vi "运维调试_采配水.vi"() -> ()   [LabVIEW 2016, in "PLC.lvlib"]
uses:
  PLC.lvlib
  <vilib>/Plasmionique/MB Master/MB_Master/MB_Master.lvclass
  <vilib>/Utility/miscctls.llb/LVPointTypeDef.ctl
  <vilib>/Plasmionique/MB Master/MB_Master_Serial/MB_Master_Serial.lvclass
  C:/Program Files (x86)/National Instruments/LabVIEW 2016/vi.lib/Plasmionique/MB Master/MB_Master/MB_Master.lvclass
  <vilib>/Instr/_visa.llb/VISA Configure Serial Port (Instr).vi
  <vilib>/Plasmionique/MB Master/MB Master.lvlib
  <vilib>/ptbypt/NI_PtbyPt.lvlib
panel:
  out "R44":i16
  in  "V14":bool
  in  "看门狗启用":bool
  out "R123":i16 caption="看门狗设置"
  out "R56":i16 caption="看门狗计时器"
  in  "更新程序":bool
  out "R122":i16 caption="二级自来水清洗时间"
  out "R121":i16 caption="一级自来水清洗时间"
  out "R120":i16 caption="过滤自来水清洗时间"
  out "清洗次数":u16
  out "当前启动泵号":u16(ring) items=["1号泵", "2号泵"]
  out "R116":i16 caption="储水时间"
  in  "R113":u16(ring) caption="水箱储水水体" items=["自来水", "水样"]
  out "R112":i16 caption="二级水样池进样超时"
  in  "R111":u16(ring) caption="采配水型号" items=["常规版本", "高配版本"]
  out "数值 19":dbl
  out "数值 18":dbl
  out "数值 17":dbl
  out "数值 16":dbl
  out "数值 15":dbl
  out "数值 14":dbl
  out "数值 13":dbl
  out "数值 12":dbl
  out "数值 11":dbl
  out "数值 10":dbl
  out "数值 9":dbl
  out "数值 8":dbl
  out "数值 7":dbl
  out "数值 6":dbl
  out "数值 5":dbl
  out "数值 4":dbl
  out "数值 3":dbl
  out "数值 2":dbl
  out "数值":dbl
  in  "R118":u16(ring) caption="是否启用质控" items=["不启用质控", "启用质控"]
  out "压力传感器":dbl format="%#.2f"
  out "R110":i16 caption="过滤装置排液时间"
  in  "M4":bool
  in  "M3":bool
  in  "V13":bool
  in  "V12":bool
  in  "V1-R":bool
  in  "V1-G":bool
  in  "V11":bool
  in  "V10":bool
  in  "V9":bool
  in  "V8":bool
  in  "V7-R":bool
  in  "V7-G":bool
  out "X2":bool caption="X1"
  out "采配水版本号":string
  out "R117":i16 caption="清洗频次设定"
  out "通讯故障":bool
  in  "R100":u16(ring) caption="采水泵工作模式" items=["泵1单泵单管路", "泵2单泵单管路", "潜水泵双泵双管路", "自吸泵双泵双管路"]
  out "X11":bool caption="自来水检测_WA"
  out "X10":bool caption="废液报警_WLA"
  out "X9":bool caption="泵2过载报警_KM2"
  out "X8":bool caption="泵1过载报警_KM1"
  out "X7":bool caption="断电检测_DD"
  out "X6":bool caption="门禁开关_MJ"
  out "X5":bool caption="烟雾检测_YW"
  out "X4":bool caption="浸水检测_SJ"
  out "X3":bool caption="水流开关_JY"
  out "X1":bool
  out "X0":bool caption="采样池液位开关_YE1"
  out "R109":i16 caption="外部反冲洗时间"
  out "集成报警信息":string
  out "R108":i16 caption="进样超时时间"
  out "R107":i16 caption="进气时间"
  out "R106":i16 caption="排液时间"
  out "R105":i16 caption="配水时间"
  out "R104":i16 caption="过滤次数"
  out "R103":i16 caption="过滤配水时间"
  out "R102":i16 caption="一级沉淀时间"
  out "R101":i16 caption="管路润洗时间"
  out "R2":i16
  out "R1":i16
  out "多列列表框":i32(listbox)
  in  "V6":bool
  in  "V5":bool
  in  "V4":bool
  in  "V3":bool
  in  "V2":bool
  in  "M2":bool
  in  "M1":bool
  in  "返回":bool
  in  "参数设置":bool
  in  "单步启动":bool
  in  "启动":bool
  in  "停止":bool
  # "流程计时："
  # "s"
  # "压力传感器："
  # "MPa"
  # "二级液位开关低_Y2FD"
  # "二级液位开关高_YF2H"
  # "看门狗设置"
  # "S"
  # "S"
  # "S"
  # "S"
  # "S"
  # "S"
  # "S"
  # "次"
  # "S"
  # "S"
  # "S"
  # "S"
  # "S"
  # "S"
  # "单步计时："
  # "s"
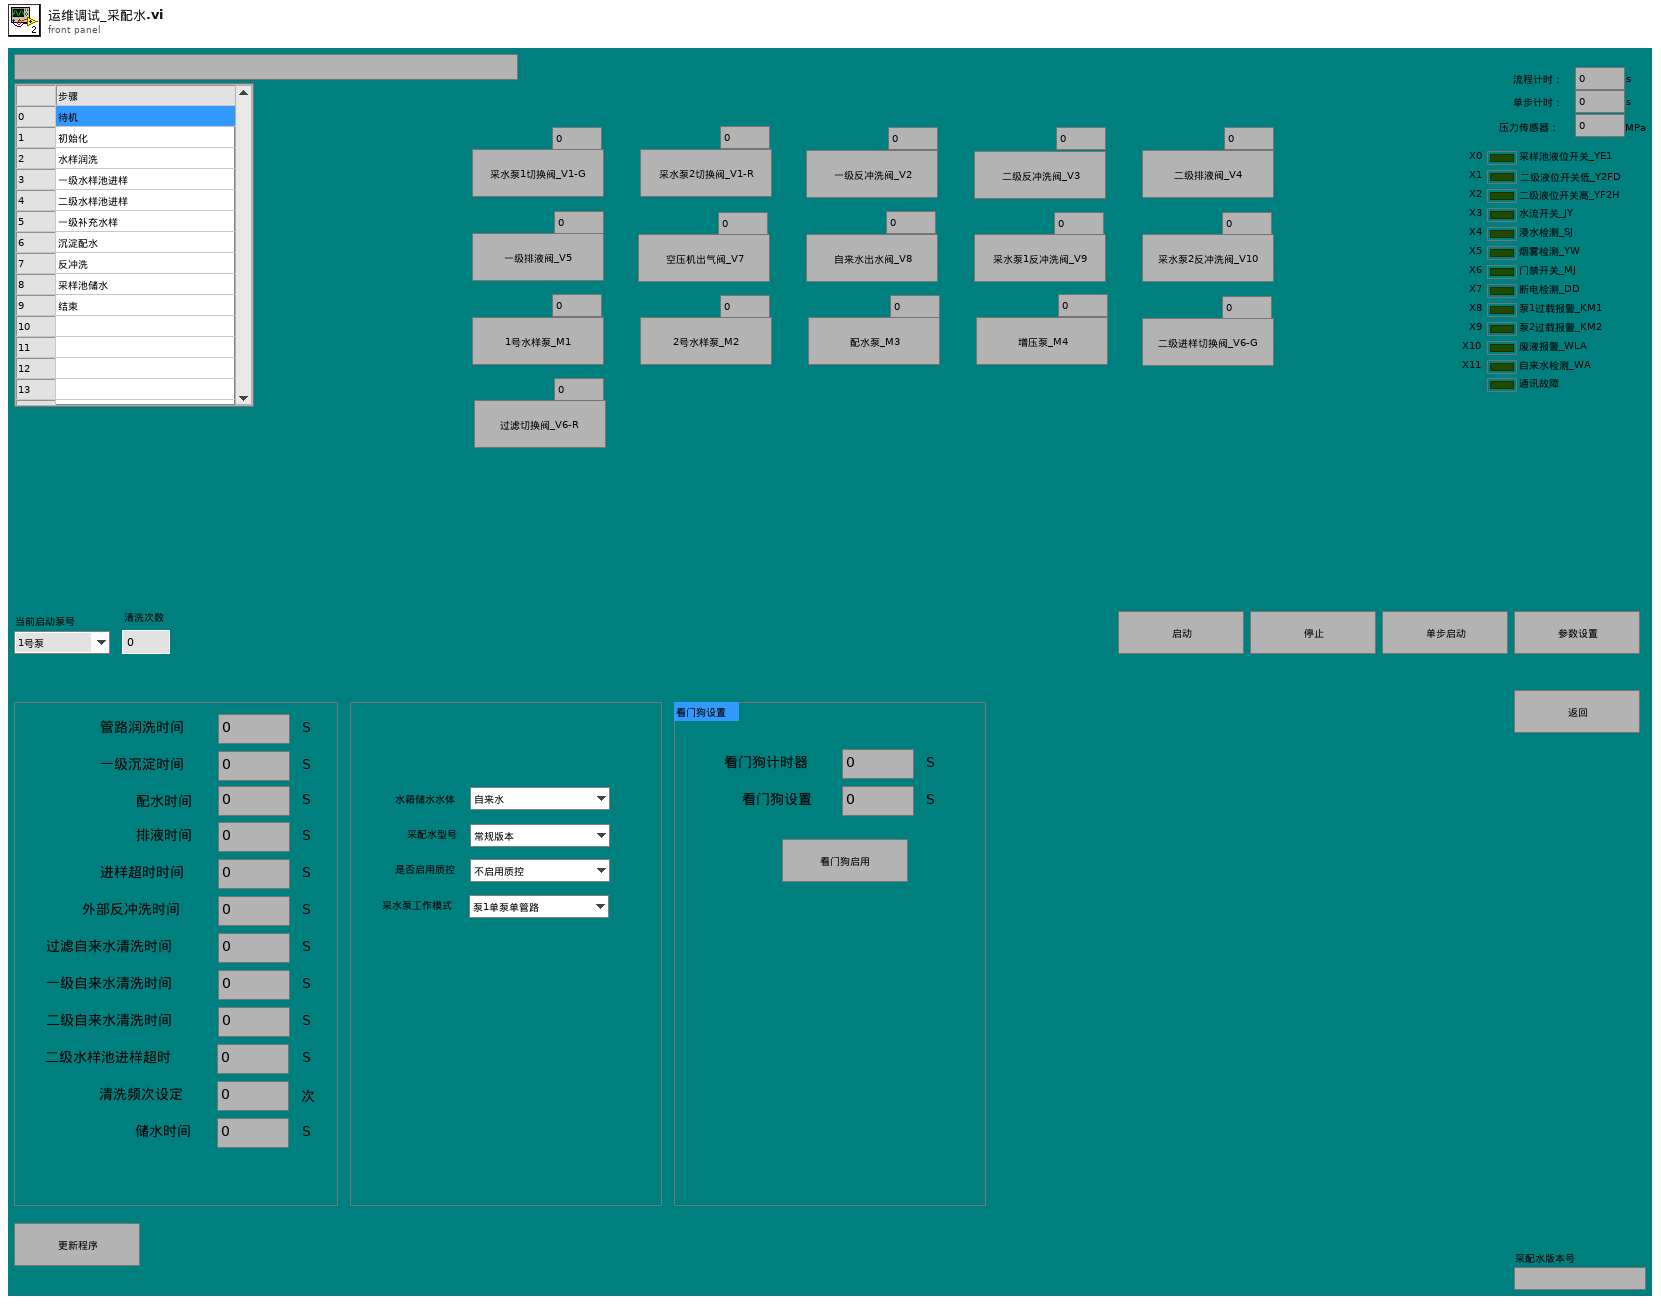
[diagram p1: front panel]
types:
  T1 = typedef "LVPointTypeDef.ctl" = cluster{"Horizontal":i16, "Vertical":i16}
  T2 = cluster{"命令":string, "数据":cluster{"starting address":u16, "holding register value":u16}}
  T3 = cluster{"时间标识":timestamp, "设备":string, "日志信息":string}
  T4 = cluster{"R0":i16, "R1":i16, "R2":i16, "R3":i16, "R4":i16, "R5":i16, "R6":i16, "R7":i16, "R8":i16, "R9":i16, "R10":i16, "R11":i16, "R12":i16, "R13":i16, "R14":i16, "R15":i16, "R16":i16, "R17":i16, "R18":i16, "R19":i16, "R20":i16, "R21":i16, "R22":i16, "R23":i16, "R24":i16, "R25":i16, "R26":i16, "R27":i16, "R28":i16, "R29":i16, "R30":i16, "R31":i16, "R32":i16, "R33":i16, "R34":i16, "R35":i16, "R36":i16, "R37":i16, "R38":i16, "R39":i16, "R40":i16, "R41":i16, "R42":i16, "R43":i16, "R44":i16, "R45":i16, "R46":i16, "R47":i16, "R48":i16, "R49":i16, "R50":i16, "R51":i16, "R52":i16, "R53":i16, "R54":i16, "R55":i16, "R56":i16}
  T5 = cluster{"seconds since 1Jan1904":timestamp, "table输入":string, string, "table输入":string}
  T6 = cluster{"时间标识":timestamp, "设备":string, "日志信息":string, "流程参数":string}
  T7 = cluster{"命令":string, cluster{"starting address":u16, "holding register value":u16}}
  T8 = cluster{"命令":string, "数据":cluster{"starting address":u16, "holding register values":u16[]}}
  T9 = cluster{"命令":string, "data":cluster{"starting address":u16, "coil values":bool[]}}
  T10 = cluster{"测试模式":enum16{"正常测试", "集成干预"}, "参数启用":cluster{"氨氮":bool, "总磷总氮":bool, "CODMn":bool, "CODcr":bool, "多参数":bool}}
  T11 = enum32{"Bad", "Idle", "Run top level", "Running"}
  T12 = cluster{"baud rate (bps)":u32, "stop bits":u16, "parity":u16, "flow control":u16, "timeout":u32, "retries":i32}
  T13 = cluster{"starting address":u16, "holding register values":u16[]}
  T14 = cluster{"starting address":u16, "holding register value":u16}
  T15 = cluster{"starting address":u16, "coil values":bool[]}
  T16 = cluster{"Registers[0]":u16, "Registers[1]":u16, "Registers[2]":u16, "Registers[3]":u16, "Registers[4]":u16, "Registers[5]":u16, "Registers[6]":u16, "Registers[7]":u16, "Registers[8]":u16, "Registers[9]":u16, "Registers[10]":u16, "Registers[11]":u16, "Registers[12]":u16, "Registers[13]":u16, "Registers[14]":u16, "Registers[15]":u16, "Registers[16]":u16, "Registers[17]":u16, "Registers[18]":u16, "Registers[19]":u16, "Registers[20]":u16, "Registers[21]":u16, "Registers[22]":u16, "Registers[23]":u16, "Registers[24]":u16, "Registers[25]":u16, "Registers[26]":u16, "Registers[27]":u16, "Registers[28]":u16, "Registers[29]":u16, "Registers[30]":u16, "Registers[31]":u16, "Registers[32]":u16, "Registers[33]":u16, "Registers[34]":u16, "Registers[35]":u16, "Registers[36]":u16, "Registers[37]":u16, "Registers[38]":u16, "Registers[39]":u16, "Registers[40]":u16, "Registers[41]":u16, "Registers[42]":u16, "Registers[43]":u16, "Registers[44]":u16, "Registers[45]":u16, "Registers[46]":u16, "Registers[47]":u16, "Registers[48]":u16, "Registers[49]":u16, "Registers[50]":u16, "Registers[51]":u16, "Registers[52]":u16, "Registers[53]":u16, "Registers[54]":u16, "Registers[55]":u16, "Registers[56]":u16}
  T17 = cluster{"Registers[0]":u16, "Registers[1]":u16, "Registers[2]":u16, "Registers[3]":u16, "Registers[4]":u16, "Registers[5]":u16}
  T18 = cluster{"Registers[0]":u16, "Registers[1]":u16, "Registers[2]":u16, "Registers[3]":u16, "Registers[4]":u16, "Registers[5]":u16, "Registers[6]":u16, "Registers[7]":u16, "Registers[8]":u16, "Registers[9]":u16, "Registers[10]":u16, "Registers[11]":u16, "Registers[12]":u16, "Registers[13]":u16, "Registers[14]":u16, "Registers[15]":u16, "Registers[16]":u16, "Registers[17]":u16, "Registers[18]":u16, "Registers[19]":u16, "Registers[20]":u16, "Registers[21]":u16, "Registers[22]":u16, "Registers[23]":u16}
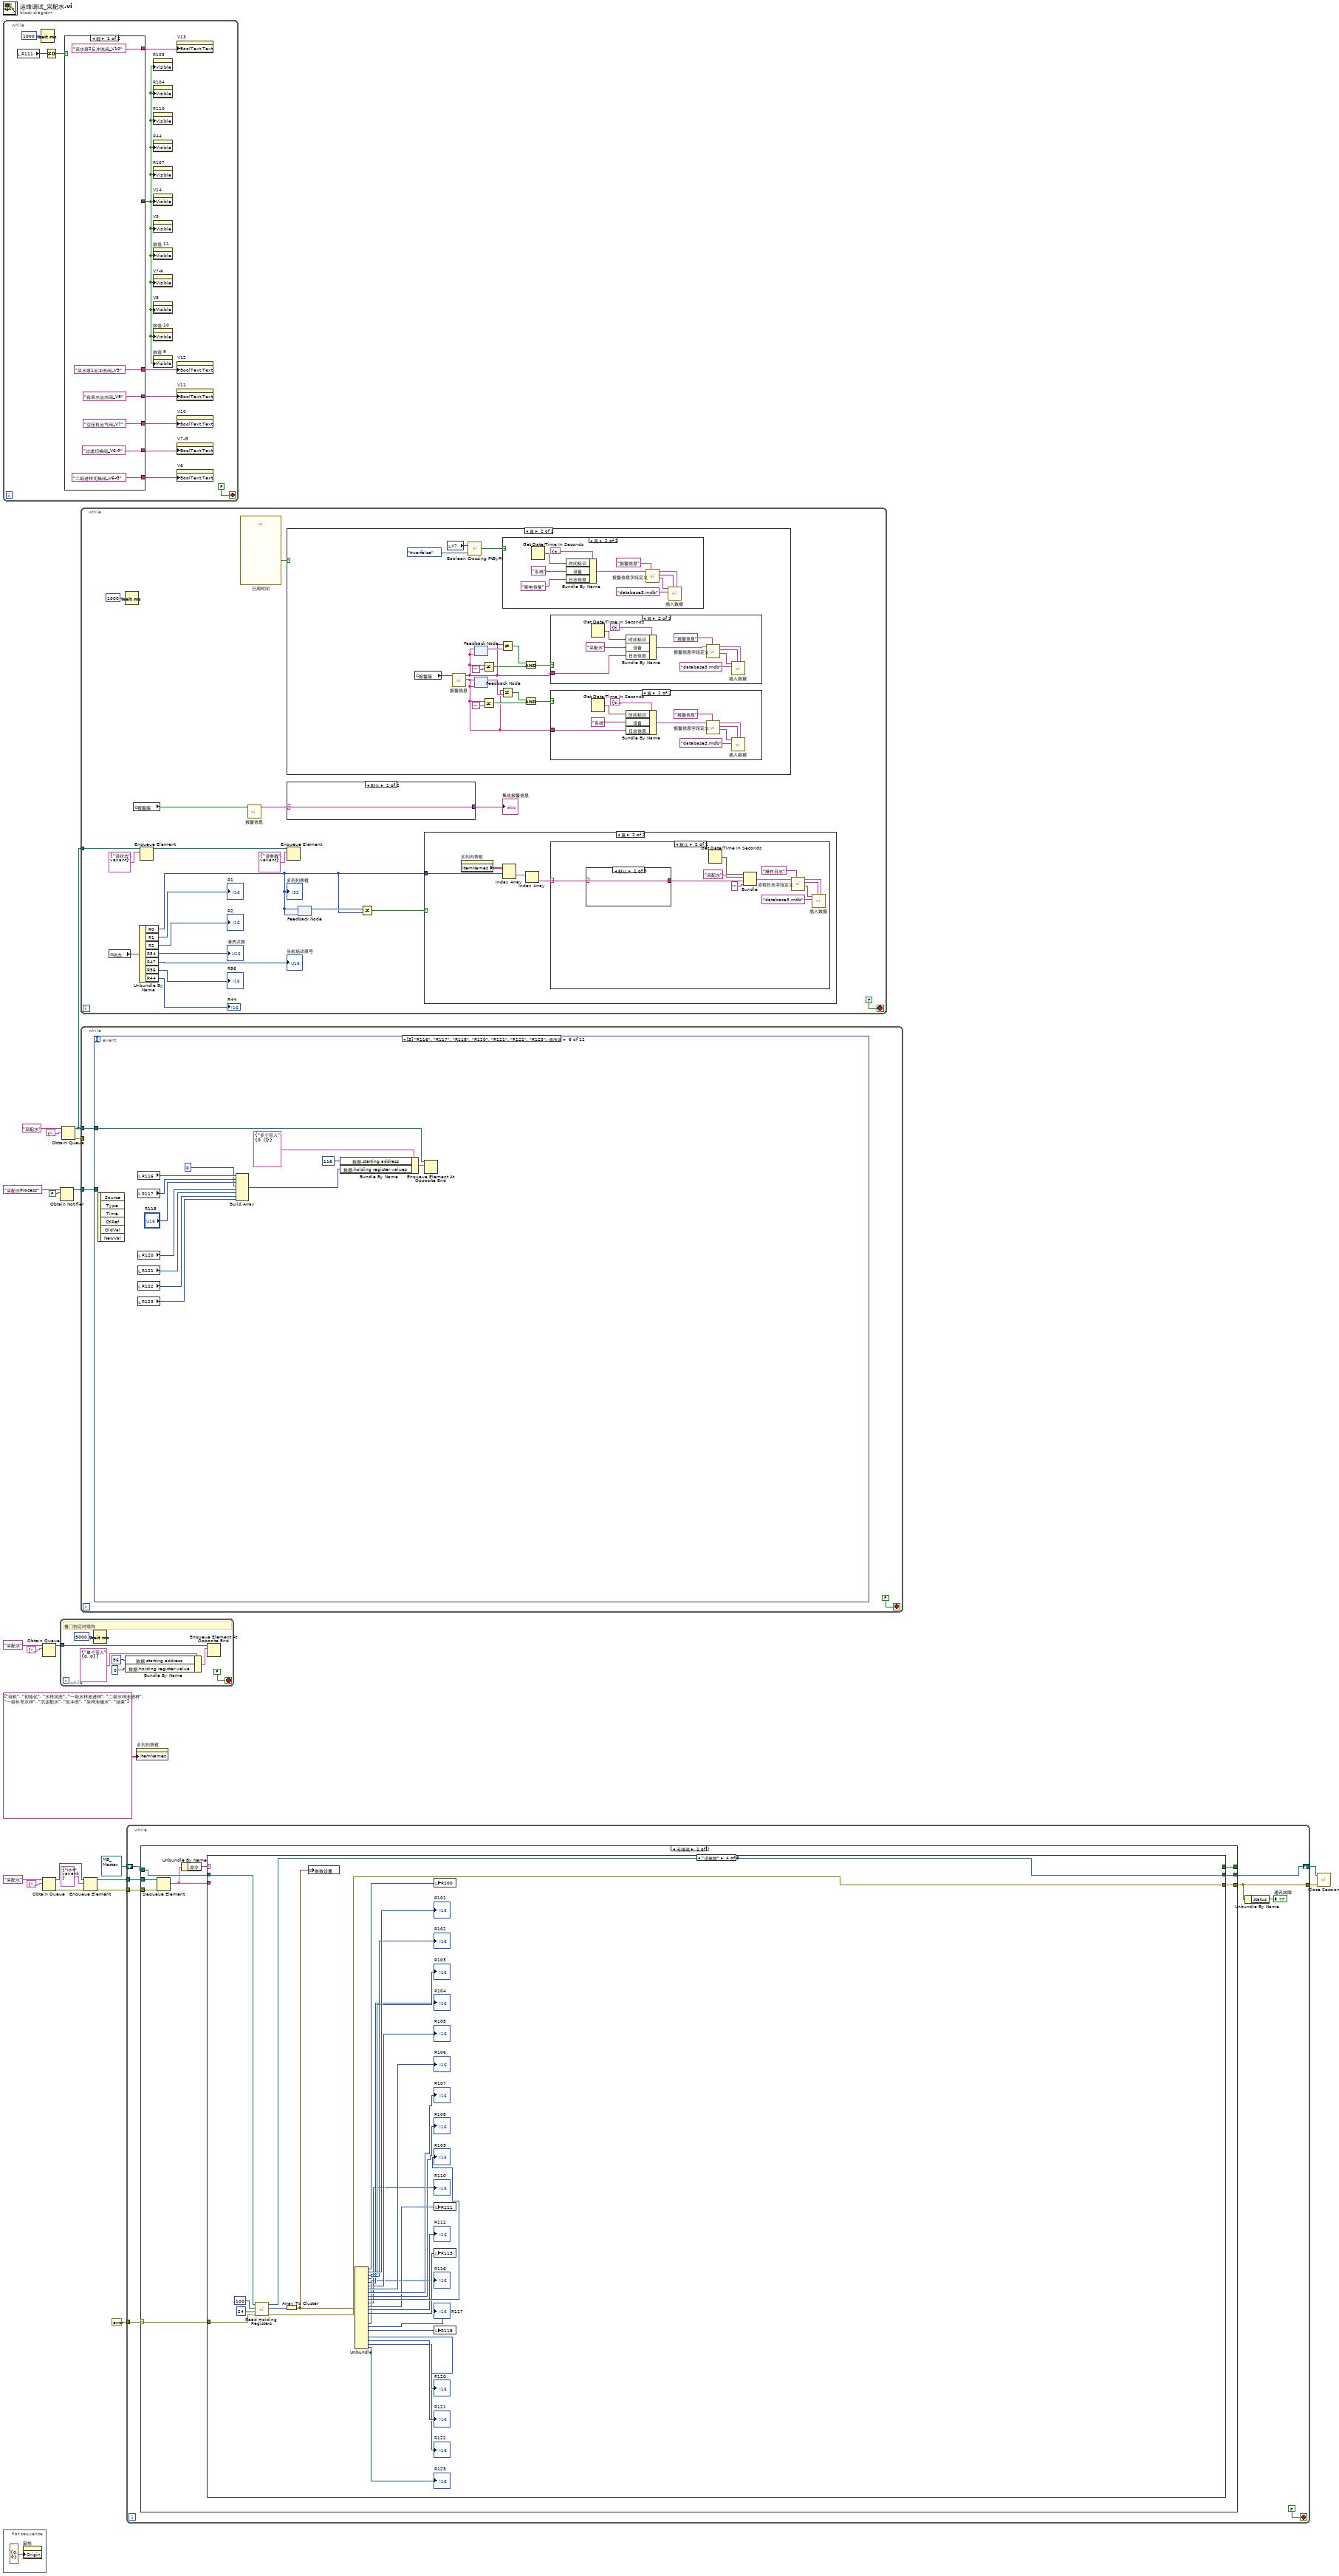
[diagram p0: block diagram]
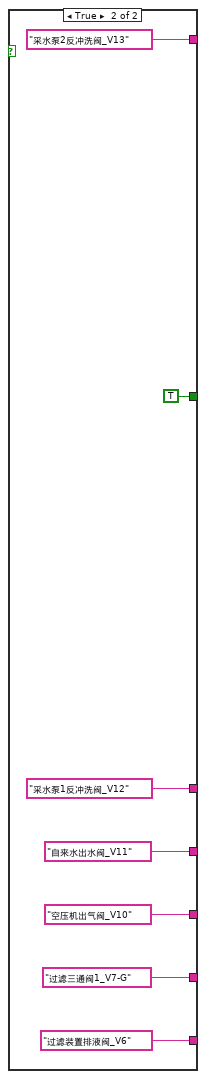
[diagram p2: hidden frame]
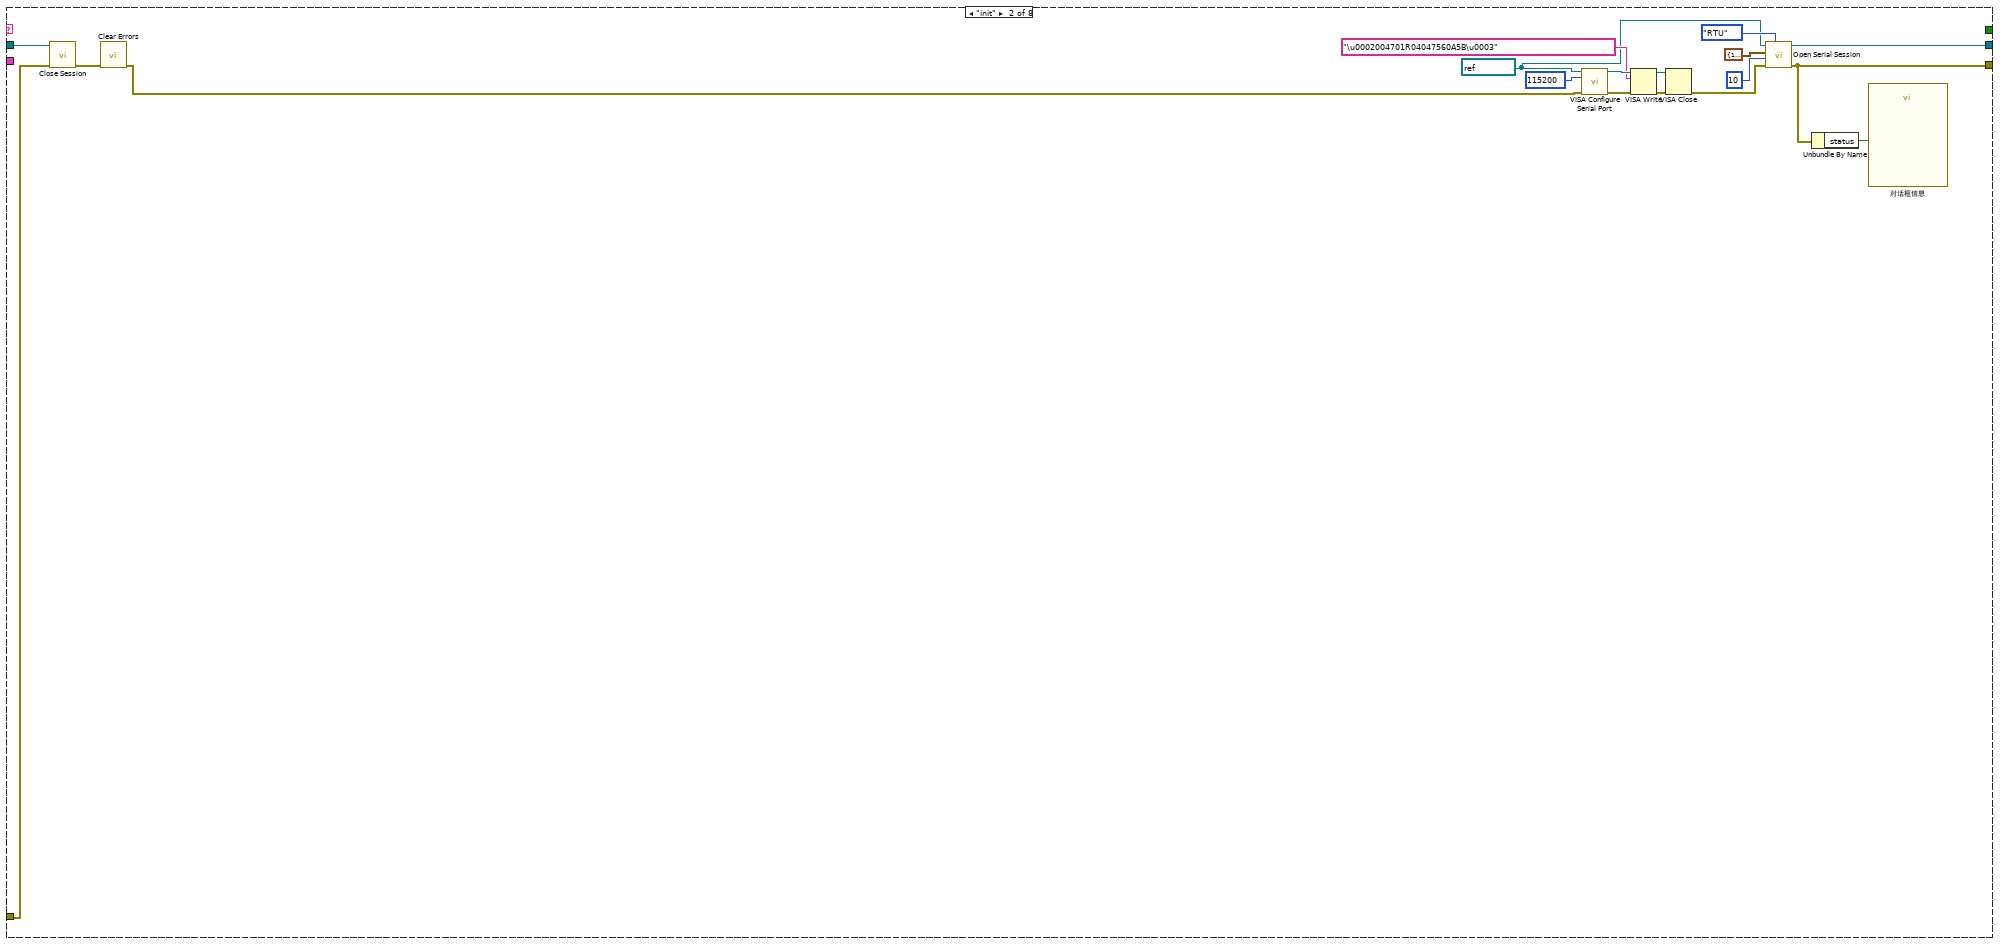
[diagram p4: hidden frame]
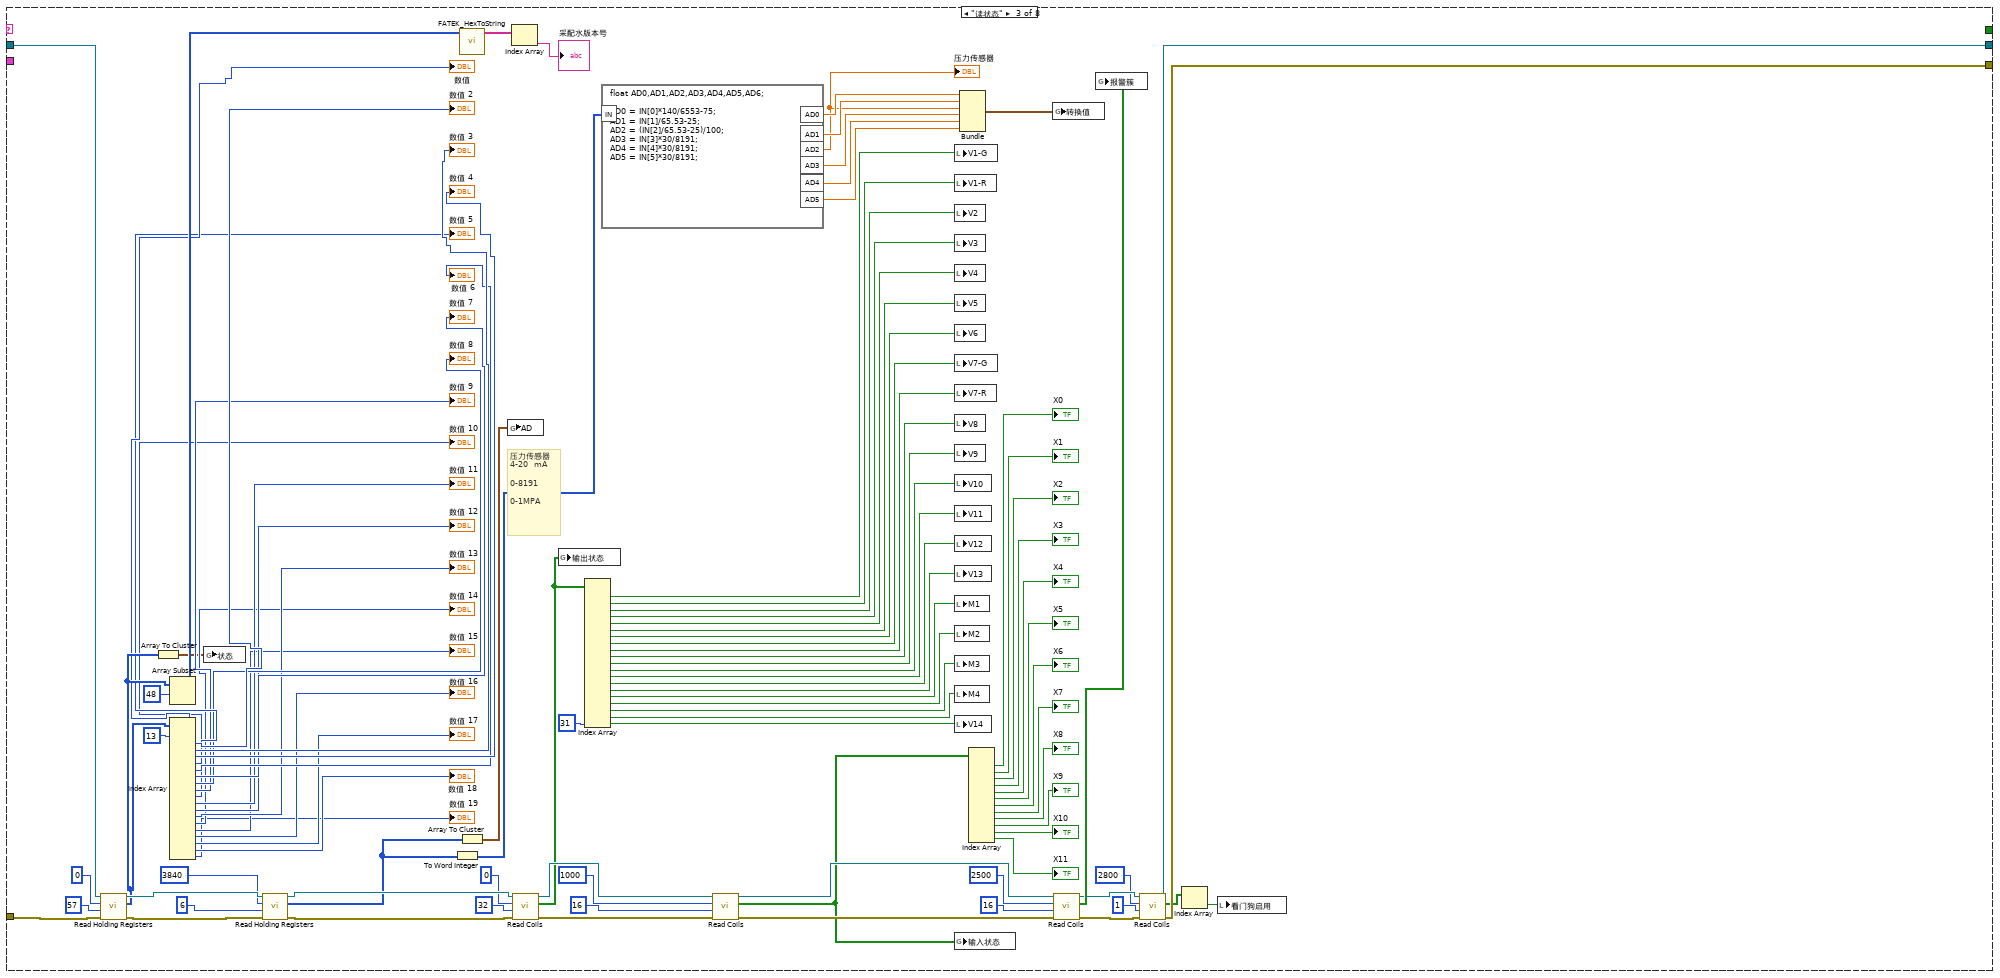
[diagram p5: hidden frame]
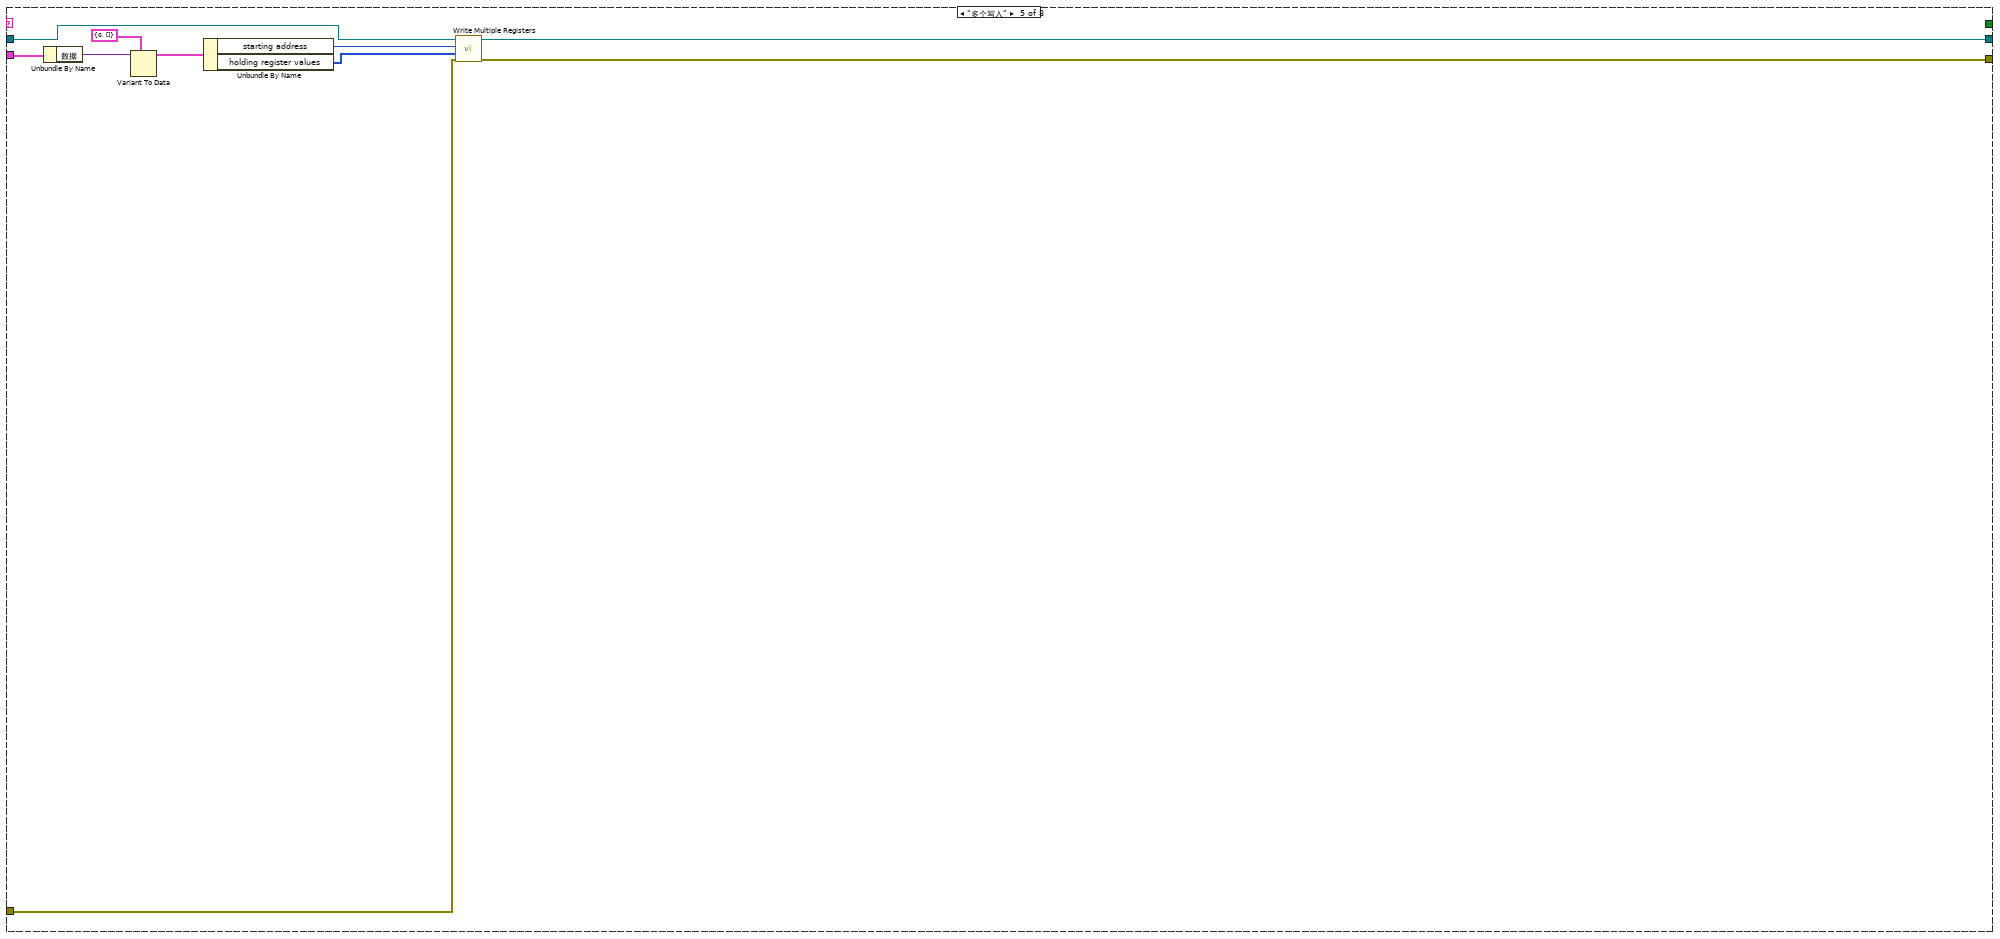
[diagram p6: hidden frame]
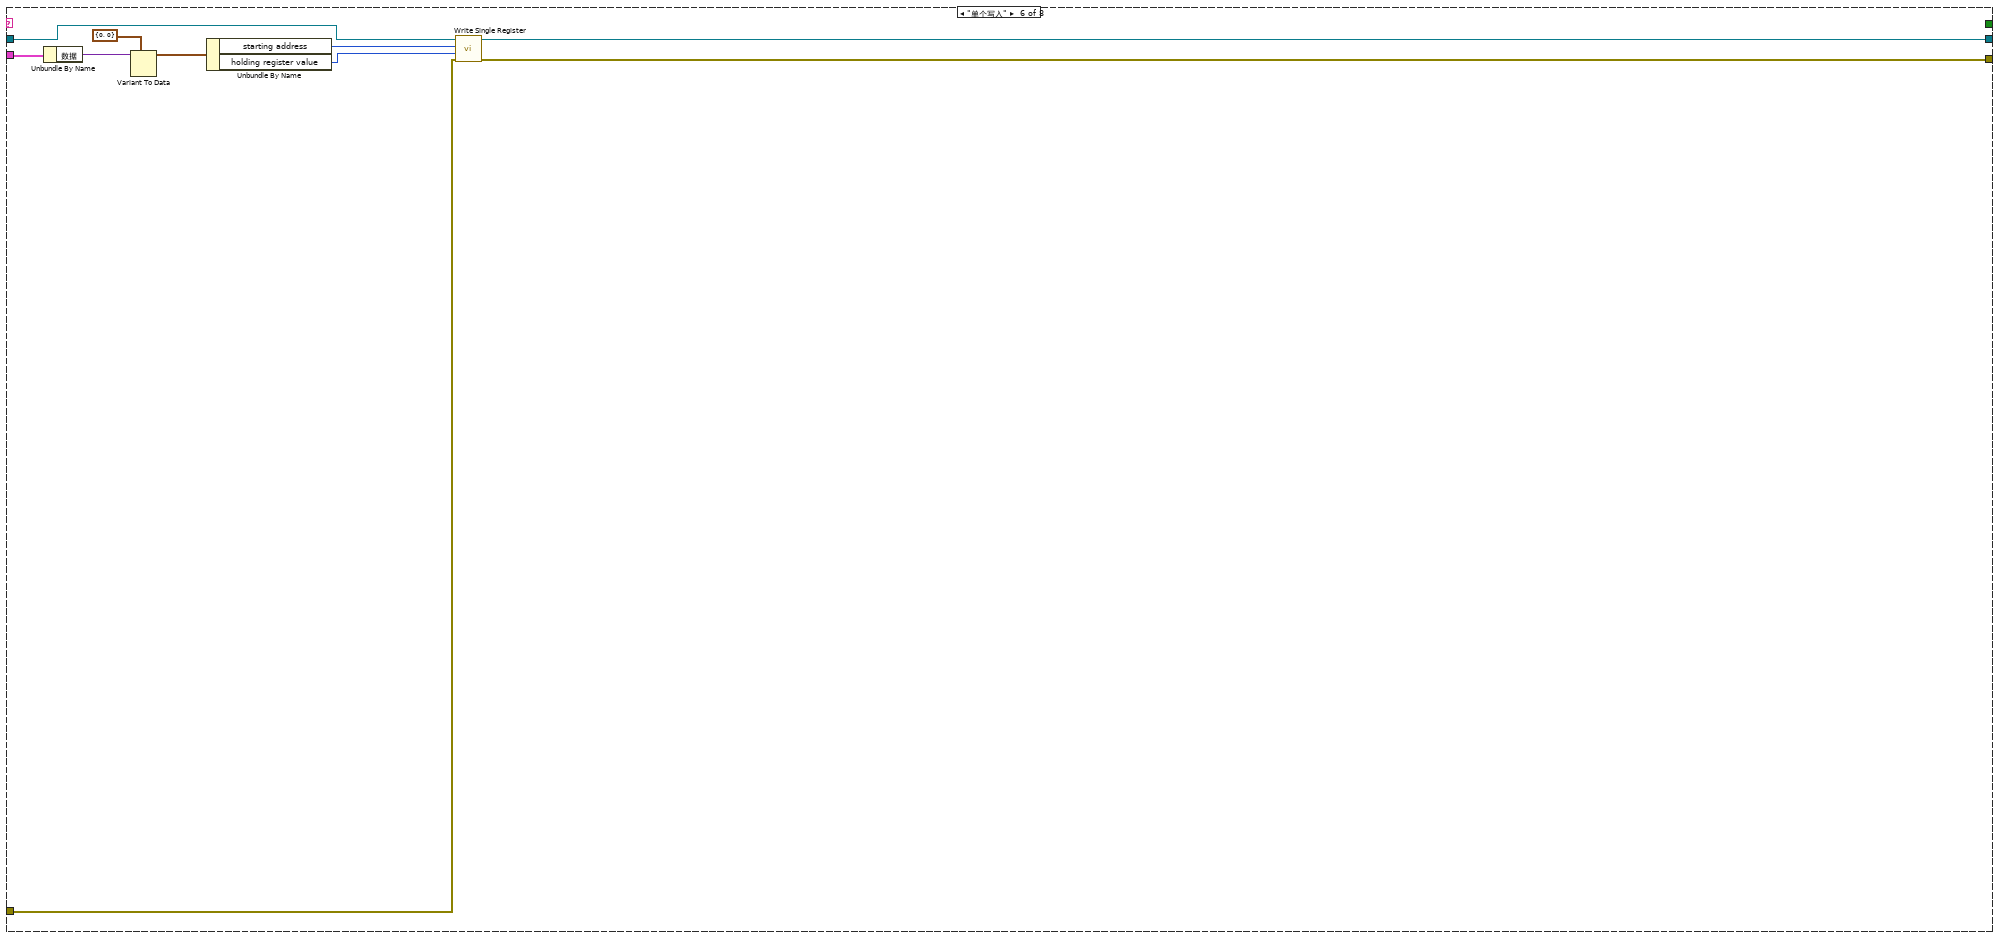
[diagram p7: hidden frame]
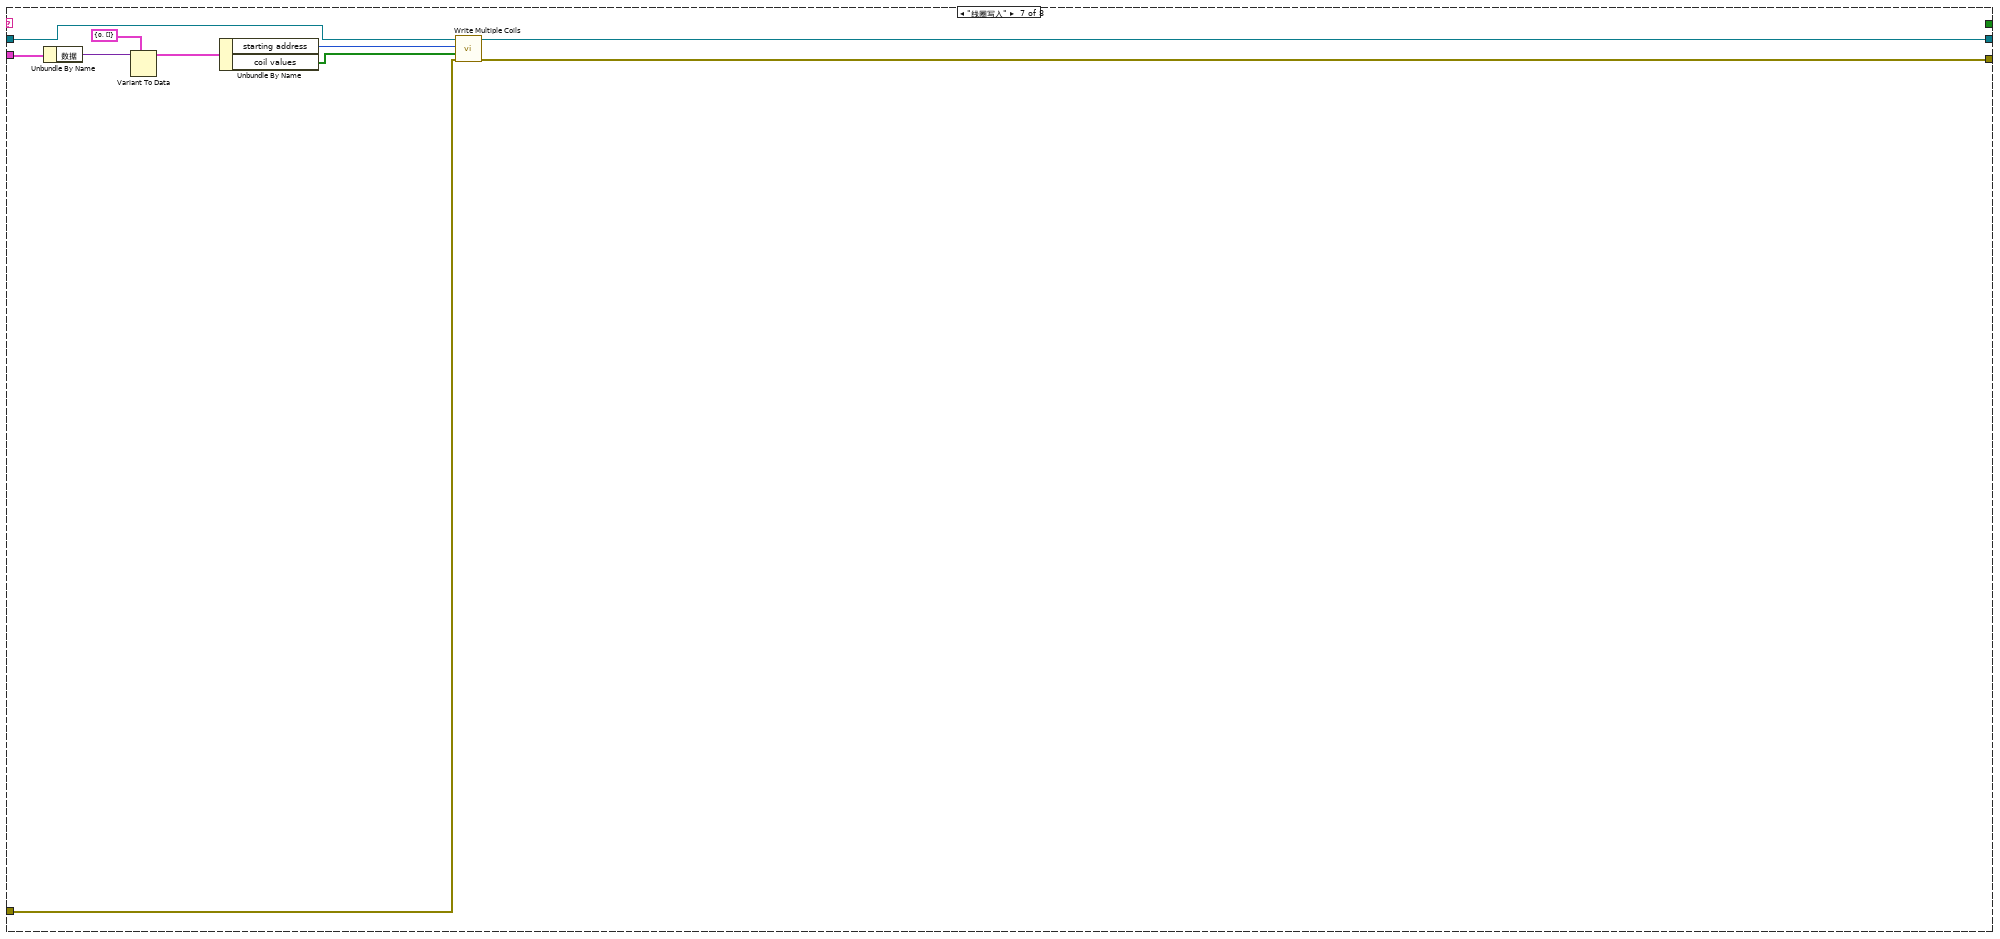
[diagram p8: hidden frame]
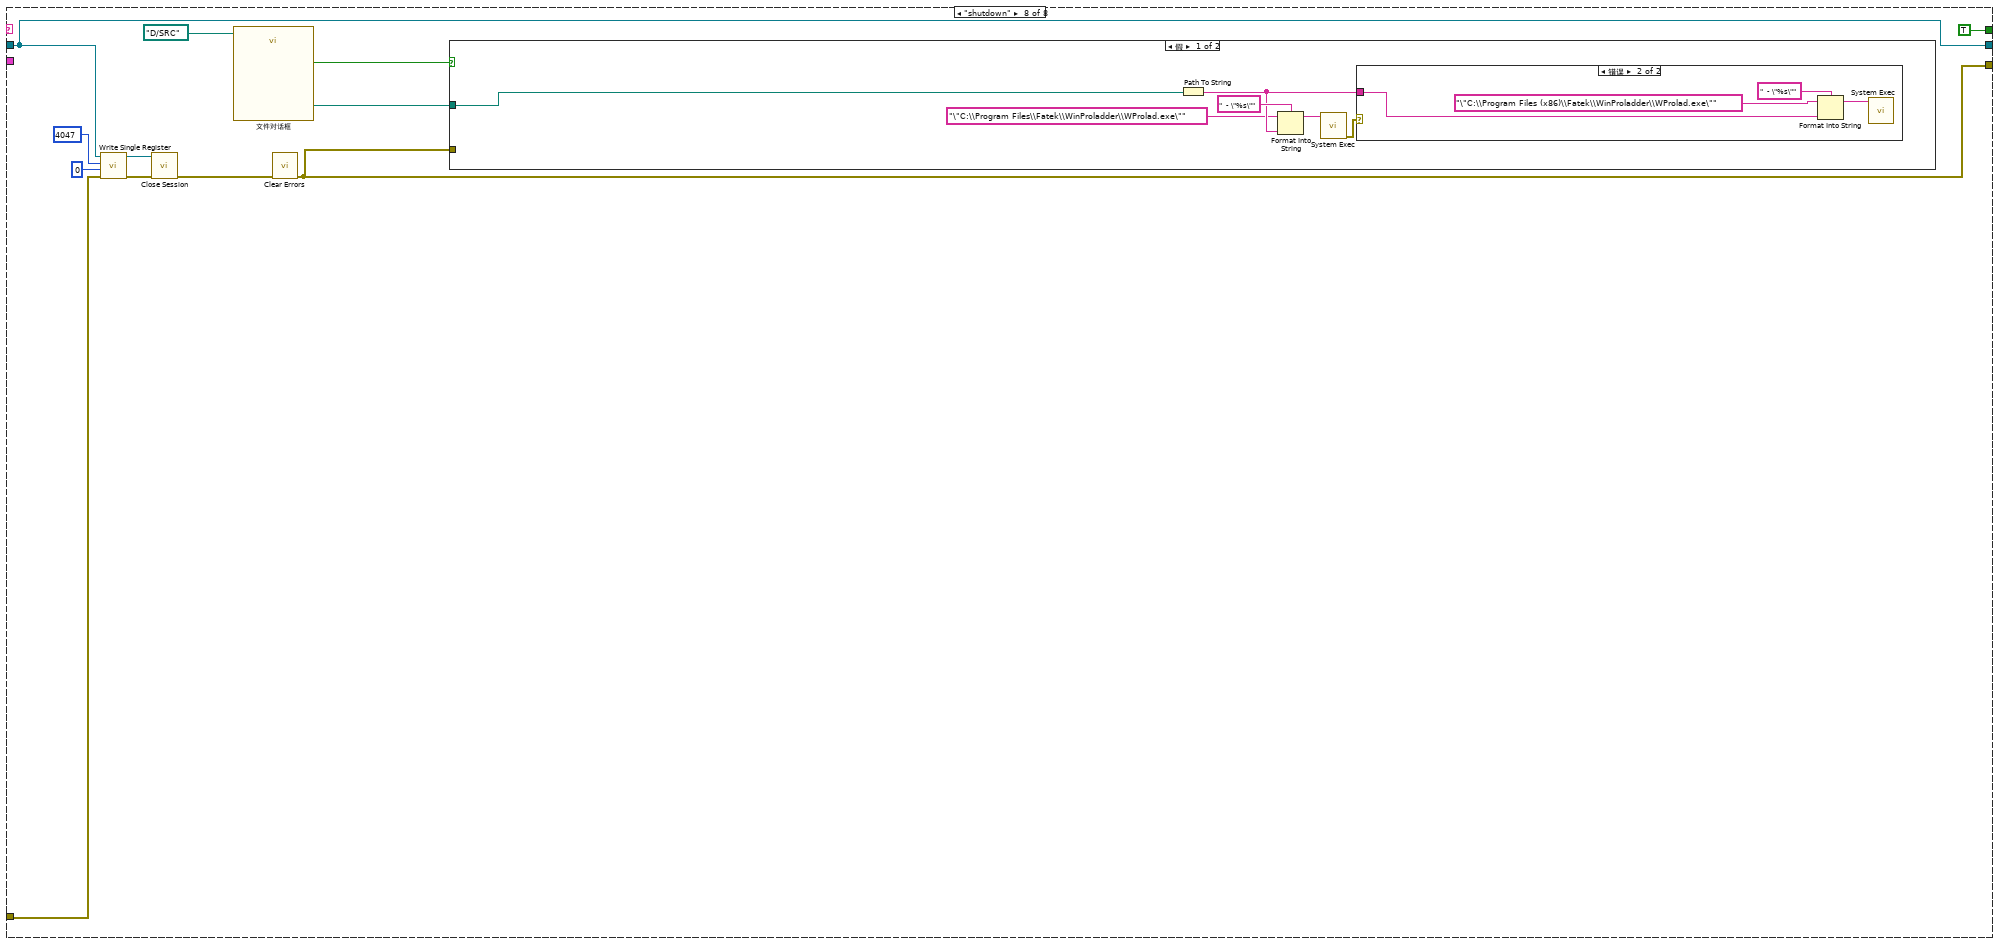
[diagram p9: hidden frame]
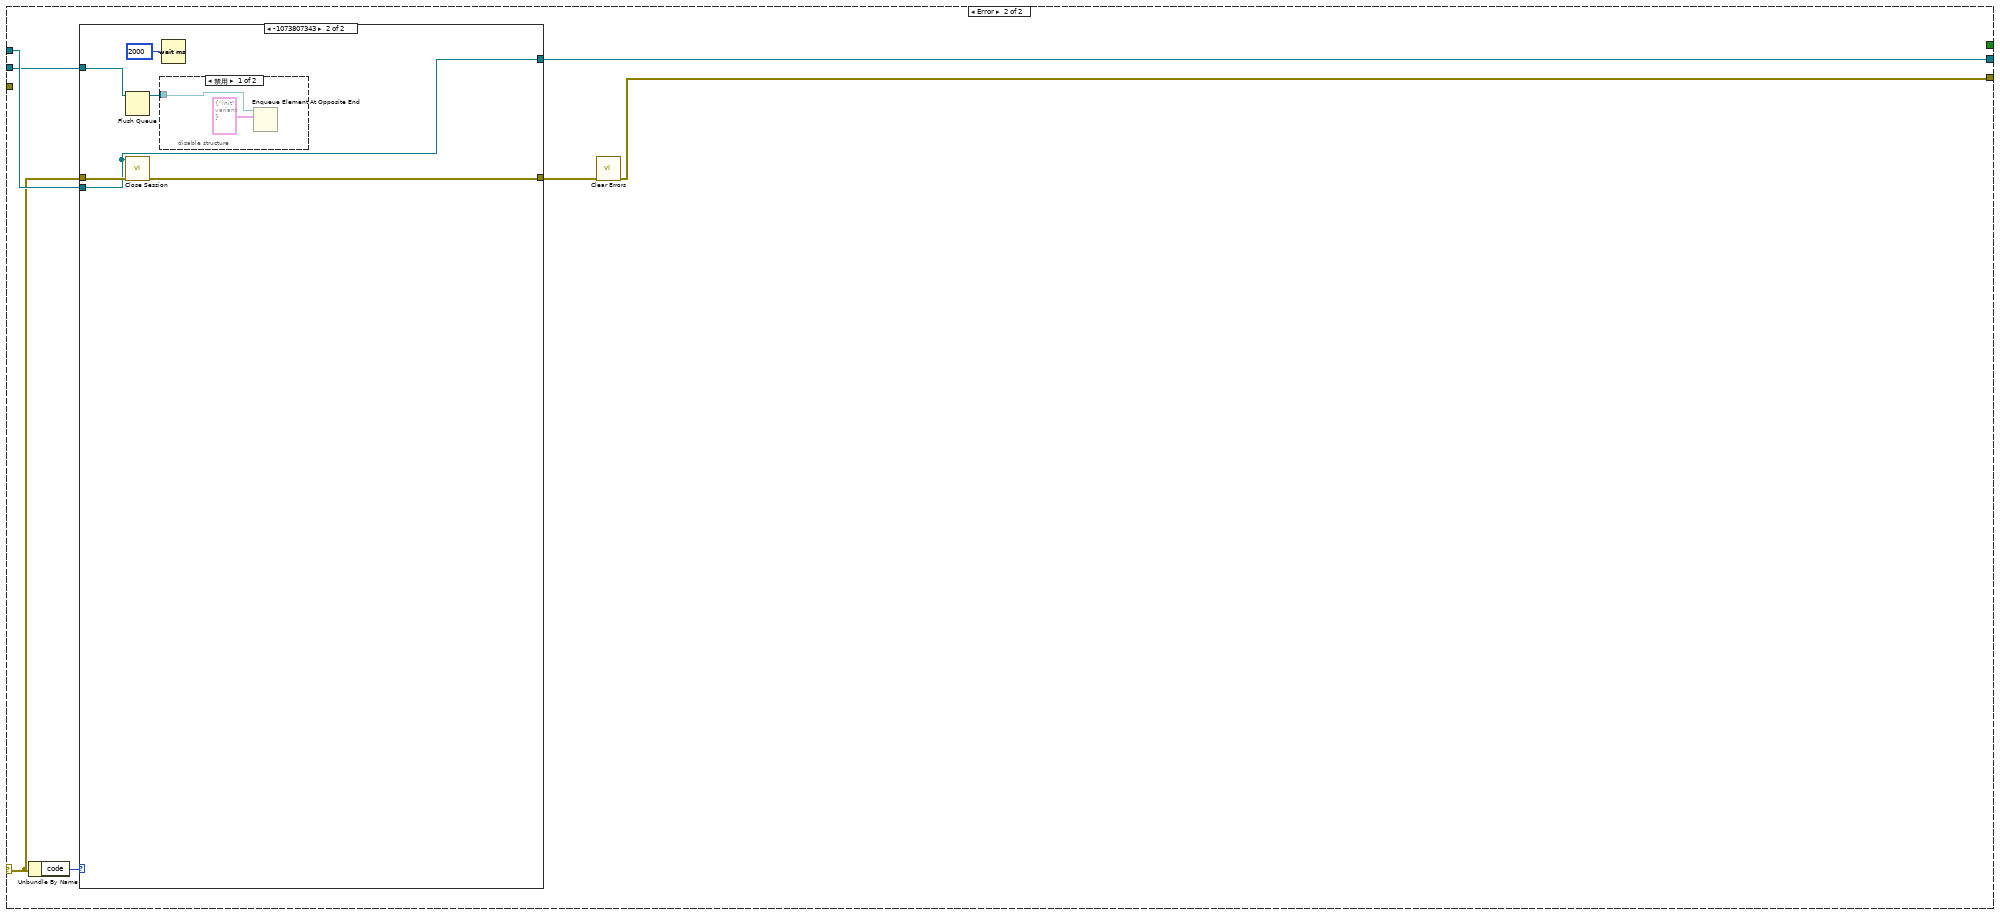
[diagram p12: hidden frame]
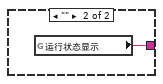
[diagram p19: hidden frame]
diagram:
  n1 = while {
    stop <- FALSE stop-if-true
    n2 = local read "R111"() -> (w32:u16)
    n3 = Wait (ms)(milliseconds to wait=u32 1000 ("等待时间（毫秒）")) -> ()  [unwired: 1 out]
    n4 = Not Equal To 0?(x=w32) -> (x != 0?=w31:bool)
    n5 = case shown="假" w31 {
      tunnel: [_ TRUE ("可见")] -> w23
      tunnel: ["二级进样切换阀_V6-G" ("布尔文本.文本") "过滤装置排液阀_V6" ("布尔文本.文本")] -> w29
      tunnel: ["过滤切换阀_V6-R" ("布尔文本.文本") "过滤三通阀1_V7-G" ("布尔文本.文本")] -> w28
      tunnel: ["空压机出气阀_V7" ("布尔文本.文本") "空压机出气阀_V10" ("布尔文本.文本")] -> w27
      tunnel: ["自来水出水阀_V8" ("布尔文本.文本") "自来水出水阀_V11" ("布尔文本.文本")] -> w26
      tunnel: ["采水泵1反冲洗阀_V9" ("布尔文本.文本") "采水泵1反冲洗阀_V12" ("布尔文本.文本")] -> w25
      tunnel: ["采水泵2反冲洗阀_V10" ("布尔文本.文本") "采水泵2反冲洗阀_V13" ("布尔文本.文本")] -> w24
      frame False {
      }
      frame True {
      }
    }
    n6 = property on="R103" class="DigNum (严格)"("Visible"=w23) -> ()  [unwired: 2 in, 2 out]
    n7 = property on="R104" class="DigNum (严格)"("Visible"=w23) -> ()  [unwired: 2 in, 2 out]
    n8 = property on="R110" class="DigNum (严格)"("Visible"=w23) -> ()  [unwired: 2 in, 2 out]
    n9 = property on="R44" class="DigNum (严格)"("Visible"=w23) -> ()  [unwired: 2 in, 2 out]
    n10 = property on="R107" class="DigNum (严格)"("Visible"=w23) -> ()  [unwired: 2 in, 2 out]
    n11 = property on="V14" class="Bool (严格)"("Visible"=w23) -> ()  [unwired: 2 in, 2 out]
    n12 = property on="V9" class="Bool (严格)"("Visible"=w23) -> ()  [unwired: 2 in, 2 out]
    n13 = property on="数值 11" class="DigNum (严格)"("Visible"=w23) -> ()  [unwired: 2 in, 2 out]
    n14 = property on="V7-R" class="Bool (严格)"("Visible"=w23) -> ()  [unwired: 2 in, 2 out]
    n15 = property on="V8" class="Bool (严格)"("Visible"=w23) -> ()  [unwired: 2 in, 2 out]
    n16 = property on="数值 10" class="DigNum (严格)"("Visible"=w23) -> ()  [unwired: 2 in, 2 out]
    n17 = property on="数值 9" class="DigNum (严格)"("Visible"=w23) -> ()  [unwired: 2 in, 2 out]
    n18 = property on="V13" class="Bool (严格)"("BoolText.Text"=w24) -> ()  [unwired: 2 in, 2 out]
    n19 = property on="V12" class="Bool (严格)"("BoolText.Text"=w25) -> ()  [unwired: 2 in, 2 out]
    n20 = property on="V11" class="Bool (严格)"("BoolText.Text"=w26) -> ()  [unwired: 2 in, 2 out]
    n21 = property on="V10" class="Bool (严格)"("BoolText.Text"=w27) -> ()  [unwired: 2 in, 2 out]
    n22 = property on="V7-G" class="Bool (严格)"("BoolText.Text"=w28) -> ()  [unwired: 2 in, 2 out]
    n23 = property on="V6" class="Bool (严格)"("BoolText.Text"=w29) -> ()  [unwired: 2 in, 2 out]
  }
  n24 = flat-sequence {
    frame #0 {
      n25 = property on="窗格" class="Pane"("Origin"=T1 {"Horizontal"=0, "Vertical"=0} ("原点")) -> ()  [unwired: 2 in, 2 out]
    }
  }
  n26 = Obtain Queue(name (unnamed)="采配水" ("名称（未命名）"), element data type=cluster{"命令":string, "数据":variant} {"命令"="", "数据"=variant}) -> (queue out=w1:refnum<queue>)  [unwired: 3 in, 2 out]
  n27 = Obtain Queue(name (unnamed)="采配水" ("名称（未命名）"), element data type=cluster{"命令":string, "数据":variant} {"命令"="", "数据"=variant}) -> (queue out=w12:refnum<queue>, error out=w11:errorcluster)  [unwired: 3 in, 1 out]
  n28 = Obtain Notifier(name (unnamed)="采配水Process" ("名称（未命名）"), notification data type=FALSE) -> (notifier out=w15:refnum<notifier>)  [unwired: 2 in, 2 out]
  n29 = while {
    tunnel: w1 -> [w52]
    stop <- FALSE stop-if-true
    # "看门狗定时喂狗"
    n30 = Wait (ms)(milliseconds to wait=u32 5000 ("等待时间（毫秒）")) -> ()  [unwired: 1 out]
    n31 = Bundle By Name(cluster=T2 {"命令"="单个写入", "数据"={"starting address"=0, "holding register value"=0}} ("元素"), "数据.starting address"=u16 56, "数据.holding register value"=u16 0) -> (w53:T2)
    n32 = Enqueue Element At Opposite End(queue=w52, element=w53) -> ()  [unwired: 2 in, 3 out]
  }
  n33 = Obtain Queue(name (unnamed)="采配水" ("名称（未命名）"), element data type=cluster{"命令":string, "数据":variant} {"命令"="", "数据"=variant}) -> (queue out=w19:refnum<queue>, error out=w20:errorcluster)  [unwired: 3 in, 1 out]
  n34 = while {
    tunnel: w19 -> [w73]
    stop <- FALSE stop-if-true
    n35 = global read "采配水全局变量.vi" "状态"() -> (w71:T4)
    n36 = Wait (ms)(milliseconds to wait=u32 1000 ("等待时间（毫秒）")) -> ()  [unwired: 1 out]
    n37 = global read "采配水全局变量.vi" "报警簇"() -> (w67:bool[])
    n38 = Unbundle By Name(w71) -> ("R0"=w60:i16, "R1"=→"R1":i16, "R2"=→"R2":i16, "R54"=→"清洗次数":i16, "R47"=→"当前启动泵号":i16, "R56"=→"R56":i16, "R44"=→"R44":i16)
    "多列列表框" <- w60
    n39 = Enqueue Element(queue=w73, element=cluster{"命令":string, "数据":variant} {"命令"="读状态", "数据"=variant} ("元素")) -> (queue out=w62:refnum<queue>)  [unwired: 2 in, 2 out]
    n40 = call "已用时间"() -> ("Time has Elapsed"=w65:bool)  [unwired: 12 in, 7 out]
    n41 = call "报警信息.vi"("报警簇"=w67) -> ("采配水报警信息"=w59:string)  [unwired: 9 in, 1 out]
    n42 = case shown="真" w65 {
      frame False {
      }
      frame True {
        n43 = global read "采配水全局变量.vi" "报警簇"() -> (w90:bool[])
        n44 = local read "X7"() -> (w77:bool)
        n45 = call "报警信息.vi"("报警簇"=w90) -> ("系统报警信息"=w79:string, "采配水报警信息"=w86:string)  [unwired: 9 in]
        n46 = call <vilib>:"Boolean Crossing PtByPt.vi"("direction"=enum16{"either", "false-true", "true-false"}."true-false", "input"=w77) -> ("crossing"=w75:bool)  [unwired: 1 in]
        n47 = feedback #1(w86) -> (w89:string)
        n48 = feedback-in #1(w86) -> ()
        n49 = feedback #2(w79) -> (w80:string)
        n50 = feedback-in #2(w79) -> ()
        n51 = Not Equal?(x=w86, y="") -> (x != y?=w84:bool)
        n52 = Not Equal?(x=w79, y="") -> (x != y?=w83:bool)
        n53 = Not Equal?(x=w86, y=w89) -> (x != y?=w88:bool)
        n54 = Not Equal?(x=w79, y=w80) -> (x != y?=w81:bool)
        n55 = case shown="真" w75 {
          frame False {
          }
          frame True {
            n56 = Get Date/Time In Seconds() -> (seconds since 1Jan1904=w99:timestamp)
            n57 = Bundle By Name(cluster=T3 {"时间标识"=timestamp(0 s since 1904-01-01), "设备"="", "日志信息"=""} ("data in"), "时间标识"=w99, "设备"="系统", "日志信息"="断电恢复") -> (w98:T3)
            n58 = call "报警信息字段定义.vi"("table输入"="报警信息", "data in"=w98) -> ("table输出"=w94:string, "columns"=w93:string[], "data out"=w92:T3)  [unwired: 7 in]
            n59 = call "插入数据.vi"("data"=w92, "columns"=w93, "database"="database3.mdb", "table"=w94) -> ()  [unwired: 7 in, 1 out]
          }
        }
        n60 = And(x=w88, y=w84) -> (x .and. y?=w87:bool)
        n61 = And(x=w81, y=w83) -> (x .and. y?=w78:bool)
        n62 = case shown="真" w87 {
          tunnel: w86 -> [_ w111]
          frame False {
          }
          frame True {
            n63 = Get Date/Time In Seconds() -> (seconds since 1Jan1904=w113:timestamp)
            n64 = Bundle By Name(cluster=T3 {"时间标识"=timestamp(0 s since 1904-01-01), "设备"="", "日志信息"=""} ("data in"), "时间标识"=w113, "设备"="采配水", "日志信息"=w111) -> (w114:T3)
            n65 = call "报警信息字段定义.vi"("table输入"="报警信息", "data in"=w114) -> ("table输出"=w118:string, "columns"=w119:string[], "data out"=w120:T3)  [unwired: 7 in]
            n66 = call "插入数据.vi"("data"=w120, "columns"=w119, "database"="database3.mdb", "table"=w118) -> ()  [unwired: 7 in, 1 out]
          }
        }
        n67 = case shown="真" w78 {
          tunnel: w79 -> [_ w101]
          frame False {
          }
          frame True {
            n68 = Get Date/Time In Seconds() -> (seconds since 1Jan1904=w103:timestamp)
            n69 = Bundle By Name(cluster=T3 {"时间标识"=timestamp(0 s since 1904-01-01), "设备"="", "日志信息"=""} ("data in"), "时间标识"=w103, "设备"="系统", "日志信息"=w101) -> (w104:T3)
            n70 = call "报警信息字段定义.vi"("table输入"="报警信息", "data in"=w104) -> ("table输出"=w108:string, "columns"=w109:string[], "data out"=w110:T3)  [unwired: 7 in]
            n71 = call "插入数据.vi"("data"=w110, "columns"=w109, "database"="database3.mdb", "table"=w108) -> ()  [unwired: 7 in, 1 out]
          }
        }
      }
    }
    n72 = case shown="默认" w59 {
      selector: w59 -> [w121 _]
      tunnel: [w121 w122] -> w66
      frame Default {
      }
      frame "" {
        n73 = global read "采配水全局变量.vi" "运行状态显示"() -> (w122:string)
      }
    }
    "集成报警信息" <- w66
    n74 = Enqueue Element(queue=w62, element=cluster{"命令":string, "数据":variant} {"命令"="读参数", "数据"=variant} ("元素")) -> ()  [unwired: 2 in, 3 out]
    n75 = feedback-in #3(w60) -> ()
    n76 = feedback #3(w60) -> (w61:i16)
    n77 = Not Equal?(x=w61, y=w60) -> (x != y?=w68:bool)
    n78 = case shown="真" w68 {
      tunnel: w60 -> [_ w125]
      frame False {
      }
      frame True {
        n79 = property on="多列列表框" class="MCListbox (严格)"() -> ("ItemNames"=w126:string[][])  [unwired: 2 in, 2 out]
        n80 = Index Array(array=w126, index (row)=w125) -> (element=w124:string[])  [unwired: 1 in]
        n81 = Index Array(array=w124) -> (element=w123:string)  [unwired: 1 in]
        n82 = case shown="默认" w123 {
          selector: w123 -> [_ w128]
          frame "待机" {
          }
          frame Default {
            n83 = case shown="默认" w128 {
              selector: w128 -> [w138 _ _]
              tunnel: [w138 "-->>启动" "-->>结束"] -> w127
              frame Default {
              }
              frame "初始化" {
              }
              frame "结束" {
              }
            }
            n84 = Get Date/Time In Seconds() -> (seconds since 1Jan1904=w132:timestamp)
            n85 = Bundle("seconds since 1Jan1904"=w132, "table输入"="采配水", w127, "table输入"="") -> (w130:T5)  [unwired: 1 in]
            n86 = call "流程日志字段定义.vi"("table输入"="操作日志", "data in"=w130) -> ("table输出"=w135:string, "columns"=w136:string[], "data out"=w137:T6)  [unwired: 7 in]
            n87 = call "插入数据.vi"("data"=w137, "columns"=w136, "database"="database3.mdb", "table"=w135) -> ()  [unwired: 7 in, 1 out]
          }
        }
      }
    }
  }
  n88 = while {
    tunnel: w19 -> [w142]
    tunnel: w20 -> [_]
    tunnel: w15 -> [w141]
    stop <- FALSE stop-if-true
    n89 = event shown="[5] \"R116\", \"R117\", \"R118\", \"R120\", \"R121\", \"R122\", \"R123\": 值改变" {
      selector: _ -> [_ _ _ _ _ _ _ _ _ _ _ _]
      dyn-events: _ -> [_ _ _ _ _ _ _ _ _ _ _ _]
      timeout: _ -> [_ _ _ _ _ _ _ _ _ _ _ _]
      tunnel: w142 -> [_ w146 w149 w171 w190 w200 _ _ _ w233 w236 w242]
      tunnel: w141 -> [_ w145 w148 _ _ _ _ _ _ _ _ _]
      event Timeout {
        n90 = event-data() -> ()  [unwired: 1 in, 3 out]
      }
      event "停止": Value Change {
        n91 = event-data() -> ()  [unwired: 1 in, 6 out]
        n92 = Send Notification(notification=TRUE ("通知"), notifier=w145) -> ()  [unwired: 1 in, 2 out]
        n93 = Enqueue Element At Opposite End(queue=w146, element=T7 {"命令"="单个写入", {"starting address"=300, "holding register value"=2}} ("元素")) -> ()  [unwired: 2 in, 3 out]
      }
      event "启动": Value Change {
        n94 = event-data() -> ()  [unwired: 1 in, 6 out]
        n95 = disable-structure shown="禁用" {
          disable-tunnel: w149 -> [w167 _]
          frame Disabled {
            n96 = Enqueue Element At Opposite End(queue=w167, element=T7 {"命令"="单个写入", {"starting address"=300, "holding register value"=1}} ("元素")) -> ()  [unwired: 2 in, 3 out]
          }
          frame Enabled {
          }
        }
        n97 = flat-sequence {
          tunnel: w148 -> [w150]
          frame #0 {
            n98 = Cancel Notification(0:w150) -> ()  [unwired: 1 in, 3 out]
          }
          frame #1 {
            n99 = call "手动启动选择对话框.vi"() -> ("确定"=w152:bool, "参数"=w151:T10)  [unwired: 10 in]
            n100 = case shown="真" w152 {
              tunnel: w151 -> [_ w153]
              frame False {
              }
              frame True {
                n101 = vi-ref "PLC.lvlib:一体站流程自动启动.vi"() -> (w156:refnum<vi>)
                n102 = property class="VI"(reference=w156) -> ("Name"=w155:string, "Exec.State"=w154:T11)  [unwired: 1 in, 2 out]
                n103 = case shown="\"Idle\"" w154 {
                  tunnel: w155 -> [_ w164 _ _]
                  tunnel: w153 -> [_ w157 _ _]
                  frame "Bad", Default {
                  }
                  frame "Idle" {
                    n104 = Open VI Reference(type specifier VI Refnum (for type only)=refnum<vi> refnum, vi path=w164, options=128 ("选项")) -> (vi reference=w162:refnum<vi>, error out=w160:errorcluster)  [unwired: 3 in]
                    n105 = call-by-ref "开始异步调用"(reference=w162, error in=w160, "参数"=w157) -> (reference out=w161:refnum<vi>, error out=w159:errorcluster)  [unwired: 11 in]
                    n106 = Close Reference(reference=w161, error in (no error)=w159) -> ()  [unwired: 1 out]
                  }
                  frame "Run top level" {
                  }
                  frame "Running" {
                    n107 = One Button Dialog(message="流程已启动，无需重复启动！" ("消息")) -> ()  [unwired: 1 in, 1 out]
                  }
                }
              }
            }
          }
        }
      }
      event "单步启动": Value Change {
        n108 = event-data() -> ()  [unwired: 1 in, 6 out]
        n109 = call "单步启动对话框.vi"() -> ("单步启动步骤输出"=w168:u16)  [unwired: 11 in]
        n110 = Bundle By Name(cluster=T2 {"命令"="单个写入", "数据"={"starting address"=301, "holding register value"=0}} ("元素"), "数据.holding register value"=w168) -> (w169:T2)
        n111 = Enqueue Element At Opposite End(queue=w171, element=w169) -> ()  [unwired: 2 in, 3 out]
      }
      event "R101", "R102", "R103", "R104", "R105", "R106", "R107", "R108", "R109", "R100", "R110", "R111", "R112", "R113": Value Change {
        n112 = event-data() -> ()  [unwired: 1 in, 6 out]
        n113 = local read "R101"() -> (w186:i16)
        n114 = local read "R102"() -> (w185:i16)
        n115 = local read "R103"() -> (w184:i16)
        n116 = local read "R104"() -> (w183:i16)
        n117 = local read "R105"() -> (w182:i16)
        n118 = local read "R106"() -> (w181:i16)
        n119 = local read "R107"() -> (w180:i16)
        n120 = local read "R108"() -> (w179:i16)
        n121 = local read "R109"() -> (w177:i16)
        n122 = local read "R110"() -> (w176:i16)
        n123 = local read "R112"() -> (w173:i16)
        n124 = Build Array("R100", w186, w185, w184, w183, w182, w181, w180, w179, w177, w176, "R111", w173, "R113") -> (w175:u16[])
        n125 = Bundle By Name(cluster=T8 {"命令"="多个写入", "数据"={"starting address"=0, "holding register values"=[]}} ("元素"), "数据.starting address"=u16 100, "数据.holding register values"=w175) -> (w187:T8)
        n126 = Enqueue Element At Opposite End(queue=w190, element=w187) -> ()  [unwired: 2 in, 3 out]
      }
      event "R116", "R117", "R118", "R120", "R121", "R122", "R123": Value Change {
        n127 = event-data() -> ()  [unwired: 1 in, 6 out]
        n128 = local read "R116"() -> (w198:i16)
        n129 = local read "R117"() -> (w197:i16)
        n130 = local read "R120"() -> (w195:i16)
        n131 = local read "R121"() -> (w194:i16)
        n132 = local read "R122"() -> (w193:i16)
        n133 = local read "R123"() -> (w192:i16)
        n134 = Build Array(w198, w197, "R118", i16 0 ("R116"), w195, w194, w193, w192) -> (w199:u16[])
        n135 = Bundle By Name(cluster=T8 {"命令"="多个写入", "数据"={"starting address"=0, "holding register values"=[]}} ("元素"), "数据.starting address"=u16 116, "数据.holding register values"=w199) -> (w201:T8)
        n136 = Enqueue Element At Opposite End(queue=w200, element=w201) -> ()  [unwired: 2 in, 3 out]
      }
      event "R101", "R102", "R103", "R104", "R105", "R106", "R107", "R108", "R109", "R117", "R110", "R116", "R112", "R120", "R121", "R122", "R123": Mouse Down {
        n137 = event-data() -> ("CtlRef"=w207:refnum<vi>)  [unwired: 1 in, 7 out]
        n138 = property class="DigNum (严格)"(reference=w207) -> (reference out=w205:refnum<vi>, "Value"=w206:i16)  [unwired: 1 in, 1 out]
        n139 = call "数字键盘.vi"("OldNumber"=w206) -> ("NewNumber"=w204:sgl)
        n140 = property class="DigNum (严格)"(reference=w205, "Val(Sgnl)"=w204) -> ()  [unwired: 1 in, 2 out]
      }
      event "参数设置": Value Change {
        n141 = event-data() -> ()  [unwired: 1 in, 6 out]
        n142 = property on="窗格" class="Pane"("Origin"=T1 {"Horizontal"=0, "Vertical"=628} ("原点")) -> ()  [unwired: 2 in, 2 out]
      }
      event "返回": Value Change {
        n143 = event-data() -> ()  [unwired: 1 in, 6 out]
        n144 = property on="窗格" class="Pane"("Origin"=T1 {"Horizontal"=0, "Vertical"=0} ("原点")) -> ()  [unwired: 2 in, 2 out]
      }
      event "M1", "M2", "V2", "V3", "V4", "V5", "V6", "V7-G", "V7-R", "V8", "V9", "V10", "V11", "V1-G", "V1-R", "V12", "V13", "M4", "M3", "V14": Value Change {
        n145 = event-data() -> ()  [unwired: 1 in, 6 out]
        n146 = Build Array("V1-G", "V1-R", "V2", "V3", "V4", "V5", "V6", "V7-G", "V7-R", "V8", "V9", "V10", "V11", "V12", "V13", "M1", "M2", "M3", "M4", "V14") -> (w226:bool[])
        n147 = Bundle By Name(cluster=T9 {"命令"="线圈写入", "data"={"starting address"=2400, "coil values"=[]}} ("元素"), "data.coil values"=w226) -> (w227:T9)
        n148 = Enqueue Element(queue=w233, element=w227) -> ()  [unwired: 2 in, 3 out]
      }
      event "看门狗启用": Value Change {
        n149 = event-data() -> ("NewVal"=w235:bool)  [unwired: 1 in, 5 out]
        n150 = Build Array(w235) -> (w234:bool[])
        n151 = Bundle By Name(cluster=T9 {"命令"="线圈写入", "data"={"starting address"=2800, "coil values"=[]}} ("元素"), "data.coil values"=w234) -> (w237:T9)
        n152 = Enqueue Element(queue=w236, element=w237) -> ()  [unwired: 2 in, 3 out]
      }
      event "更新程序": Value Change {
        n153 = event-data() -> ("NewVal"=w239:bool)  [unwired: 1 in, 5 out]
        n154 = case shown="真" w239 {
          tunnel: [cluster{"命令":string, "数据":variant} {"命令"="init", "数据"=variant} ("元素") w246] -> w241
          frame False {
          }
          frame True {
            n155 = Two Button Dialog(message="警告，非专业人士请勿进行此操作！！！\n请确认是否释放串口？" ("消息")) -> (T button?=w245:bool)  [unwired: 2 in]
            n156 = case shown="真" w245 {
              tunnel: [_ cluster{"命令":string, "数据":variant} {"命令"="shutdown", "数据"=variant} ("元素")] -> w246
              frame False {
                n157 = local write "更新程序"(FALSE ("释放串口")) -> ()
              }
              frame True {
              }
            }
          }
        }
        n158 = Flush Queue(queue=w242) -> (queue out=w240:refnum<queue>)  [unwired: 1 in, 2 out]
        n159 = Enqueue Element(queue=w240, element=w241) -> ()  [unwired: 2 in, 3 out]
      }
    }
  }
  n160 = Enqueue Element(queue=w12, element=cluster{"命令":string, "数据":variant} {"命令"="init", "数据"=variant} ("元素"), error in (no error)=w11) -> (queue out=w7:refnum<queue>, error out=w9:errorcluster)  [unwired: 1 in, 1 out]
  n161 = while {
    tunnel: w7 -> [w253]
    tunnel: w9 -> [w252]
    shift-right: [w256] -> w4
    shift-left: refnum<class "MB_Master.lvclass"> refnum ("MB session in") -> [w255]
    tunnel: errorcluster {"status"=FALSE, "code"=0, "source"=""} ("error out") -> [w254]
    tunnel: [w251] -> w5
    stop <- FALSE stop-if-true
    n162 = case shown="无错误" w254 {
      selector: w254 -> [w262 w471]
      tunnel: [w265 w470] -> w256
      tunnel: w255 -> [w264 w472]
      tunnel: [w263 w468] -> w251
      tunnel: w253 -> [w259 w467]
      tunnel: w252 -> [w258 _]
      tunnel: [w260 _] -> _
      frame No Error {
        n163 = Dequeue Element(queue=w259, error in (no error)=w258) -> (element=w257:cluster{"命令":string, "数据":variant})  [unwired: 1 in, 3 out]
        n164 = Unbundle By Name(w257) -> ("命令"=w261:string)
        n165 = case shown="\"读参数\"" w261 {
          tunnel: [w267 w280 w294 w409 w421 w431 w441 w454] -> w265
          tunnel: w264 -> [w267 w282 w375 w414 w424 w434 w444 w454]
          tunnel: [w266 w281 w292 w408 w422 w432 w442 w445] -> w263
          tunnel: w262 -> [w266 w284 w378 w413 w423 w433 w443 w450]
          tunnel: [_ _ _ _ _ _ _ TRUE] -> w260
          tunnel: w257 -> [_ _ _ _ w420 w430 w440 _]
          frame "idle", Default {
          }
          frame "init" {
            w271 = refnum<visa-resource-name> "COM3" ("VISA resource name")
            n166 = call-dynamic "Close Session.vi"("error in (no error)"=w284, "MB session in"=w282) -> ("error out"=w283:errorcluster)  [unwired: 9 in]
            n167 = call <vilib>:"Clear Errors.vi"("error in (no error)"=w283) -> ("error out"=w269:errorcluster)  [unwired: 5 in, 1 out]
            n168 = call-poly "VISA Configure Serial Port"("VISA resource name"=w271, "baud rate (9600)"=u32 115200, "error in (no error)"=w269) -> ("VISA resource name out"=w276:refnum<visa-resource-name>, "error out"=w275:errorcluster)  [unwired: 11 in]
            n169 = VISA Write(VISA resource name=w276, write buffer="\u0002004701R04047560A5B\u0003" ("写入缓冲区"), error in (no error)=w275) -> (VISA resource name out=w274:refnum<visa-resource-name>, error out=w273:errorcluster)  [unwired: 1 out]
            n170 = VISA Close(VISA resource name=w274, error in (no error)=w273) -> (error out=w268:errorcluster)
            n171 = call <vilib>:"Open Serial Session.vi"("Mode (RTU)"=enum16{"RTU", "ASCII"}."RTU", "Error in"=w268, "Slave ID"=u8 10, "Serial Config"=T12 {"baud rate (bps)"=115200, "stop bits"=10, "parity"=0, "flow control"=0, "timeout"=500, "retries"=1}, "VISA Resource"=w271) -> ("Error out"=w281:errorcluster, "MB_Serial session"=w280:refnum<class "MB_Master_Serial.lvclass">)  [unwired: 5 in]
            n172 = Unbundle By Name(w281) -> ("status"=w285:bool)
            n173 = call "对话框信息"("Enable"=w285) -> ()  [unwired: 9 in, 2 out]
          }
          frame "读状态" {
            # "压力传感器\n4-20  mA \n \n0-8191\n\n0-1MPA"
            n174 = call <vilib>:"Read Holding Registers.vi"("error in (no error)"=w378, "quantity"=u16 57 ("number of holding registers"), "starting address"=u16 0, "MB session in"=w375) -> ("error out"=w373:errorcluster, "Registers"=w317:u16[], "MB session out"=w374:refnum<class "MB_Master.lvclass">)  [unwired: 5 in]
            n175 = Array To Cluster(array=w317) -> (cluster=w296:T16)
            n176 = Array Subset(array=w317, index=48 ("索引")) -> (w343:u16[])  [unwired: 1 in]
            n177 = Index Array(array=w317, index #1=13 ("索引")) -> (element #1=→"数值":u16, element #2=→"数值 2":u16, element #3=→"数值 3":u16, element #4=→"数值 4":u16, element #5=→"数值 5":u16, element #6=→"数值 6":u16, element #7=→"数值 7":u16, element #8=→"数值 8":u16, element #9=→"数值 9":u16, element #10=→"数值 10":u16, element #11=→"数值 11":u16, element #12=→"数值 12":u16, element #13=→"数值 13":u16, element #14=→"数值 14":u16, element #15=→"数值 15":u16, element #16=→"数值 16":u16, element #17=→"数值 17":u16, element #18=→"数值 18":u16, element #19=→"数值 19":u16)  [unwired: 18 in]
            n178 = global write "采配水全局变量.vi" "状态"(w296) -> ()
            n179 = call <vilib>:"Read Holding Registers.vi"("error in (no error)"=w373, "quantity"=u16 6 ("number of holding registers"), "starting address"=u16 3840, "MB session in"=w374) -> ("error out"=w369:errorcluster, "Registers"=w346:u16[], "MB session out"=w370:refnum<class "MB_Master.lvclass">)  [unwired: 5 in]
            n180 = To Word Integer(number=w346) -> (16bit integer=w345:i16[])
            n181 = call "FATEK_HexToString.vi"("数组"=w343) -> ("STRING"=w342:string[])  [unwired: 10 in]
            n182 = Array To Cluster(array=w346) -> (cluster=w385:T17)
            n183 = global write "采配水全局变量.vi" "AD"(w385) -> ()
            n184 = Index Array(array=w342) -> (element=→"采配水版本号":string)  [unwired: 1 in]
            n185 = call <vilib>:"Read Coils.vi"("error in (no error)"=w369, "quantity"=u16 32 ("number of coils"), "starting address"=u16 0, "MB session in"=w370) -> ("error out"=w365:errorcluster, "Coils"=w350:bool[], "MB session out"=w366:refnum<class "MB_Master.lvclass">)  [unwired: 5 in]
            n186 = global write "采配水全局变量.vi" "输出状态"(w350) -> ()
            n187 = Index Array(array=w350, index #20=31 ("索引")) -> (element #1=w324:bool, element #2=w340:bool, element #3=w339:bool, element #4=w338:bool, element #5=w337:bool, element #6=w336:bool, element #7=w335:bool, element #8=w331:bool, element #9=w330:bool, element #10=w329:bool, element #11=w328:bool, element #12=w327:bool, element #13=w326:bool, element #14=w323:bool, element #15=w322:bool, element #16=w321:bool, element #17=w320:bool, element #18=w319:bool, element #19=w318:bool, element #20=w286:bool)  [unwired: 19 in]
            n188 = formula code="float AD0,AD1,AD2,AD3,AD4,AD5,AD6;\n\nAD0 = IN[0]*140/6553-75;\nAD1 = IN[1]/65.53-25;\nAD2 = (IN[2]/65.53-25)/100;\nAD3 = IN[3]*30/8191;\nAD4 = IN[4]*30/8191;\nAD5 = IN[5]*30/8191;"("IN"=w345) -> ("AD0"=w383:dbl, "AD1"=w382:dbl, "AD2"=w325:dbl, "AD3"=w381:dbl, "AD4"=w380:dbl, "AD5"=w379:dbl)
            "压力传感器" <- w325
            n189 = call <vilib>:"Read Coils.vi"("error in (no error)"=w365, "quantity"=u16 16 ("number of coils"), "starting address"=u16 1000, "MB session in"=w366) -> ("error out"=w361:errorcluster, "Coils"=w357:bool[], "MB session out"=w362:refnum<class "MB_Master.lvclass">)  [unwired: 5 in]
            n190 = local write "V1-G"(w324) -> ()
            n191 = local write "V1-R"(w340) -> ()
            n192 = local write "V2"(w339) -> ()
            n193 = local write "V3"(w338) -> ()
            n194 = local write "V4"(w337) -> ()
            n195 = local write "V5"(w336) -> ()
            n196 = local write "V6"(w335) -> ()
            n197 = local write "V7-G"(w331) -> ()
            n198 = local write "V7-R"(w330) -> ()
            n199 = local write "V8"(w329) -> ()
            n200 = local write "V9"(w328) -> ()
            n201 = local write "V10"(w327) -> ()
            n202 = local write "V11"(w326) -> ()
            n203 = local write "V12"(w323) -> ()
            n204 = local write "V13"(w322) -> ()
            n205 = local write "M1"(w321) -> ()
            n206 = local write "M2"(w320) -> ()
            n207 = local write "M3"(w319) -> ()
            n208 = local write "M4"(w318) -> ()
            n209 = local write "V14"(w286) -> ()
            n210 = global write "采配水全局变量.vi" "输入状态"(w357) -> ()
            n211 = Bundle(w383, w382, w325, w381, w380, w379) -> (w384:cluster{dbl, dbl, dbl, dbl, dbl, dbl})  [unwired: 1 in]
            n212 = Index Array(array=w357) -> (element #1=→"X0":bool, element #2=→"X1":bool, element #3=→"X2":bool, element #4=→"X3":bool, element #5=→"X4":bool, element #6=→"X5":bool, element #7=→"X6":bool, element #8=→"X7":bool, element #9=→"X8":bool, element #10=→"X9":bool, element #11=→"X10":bool, element #12=→"X11":bool)  [unwired: 12 in]
            n213 = global write "采配水全局变量.vi" "转换值"(w384) -> ()
            n214 = call <vilib>:"Read Coils.vi"("error in (no error)"=w361, "quantity"=u16 16 ("number of coils"), "starting address"=u16 2500, "MB session in"=w362) -> ("error out"=w293:errorcluster, "Coils"=w358:bool[], "MB session out"=w295:refnum<class "MB_Master.lvclass">)  [unwired: 5 in]
            n215 = global write "采配水全局变量.vi" "报警簇"(w358) -> ()
            n216 = call <vilib>:"Read Coils.vi"("error in (no error)"=w293, "quantity"=u16 1, "starting address"=u16 2800, "MB session in"=w295) -> ("error out"=w292:errorcluster, "Coils"=w289:bool[], "MB session out"=w294:refnum<class "MB_Master.lvclass">)  [unwired: 5 in]
            n217 = Index Array(array=w289) -> (element=w288:bool)  [unwired: 1 in]
            n218 = local write "看门狗启用"(w288) -> ()
          }
          frame "读参数" {
            n219 = call <vilib>:"Read Holding Registers.vi"("error in (no error)"=w413, "quantity"=u16 24 ("number of holding registers"), "starting address"=u16 100, "MB session in"=w414) -> ("error out"=w408:errorcluster, "Registers"=w410:u16[], "MB session out"=w409:refnum<class "MB_Master.lvclass">)  [unwired: 5 in]
            n220 = Array To Cluster(array=w410) -> (cluster=w398:T18)
            n221 = global write "采配水全局变量.vi" "参数设置"(w398) -> ()
            n222 = Unbundle(w398) -> ("Registers[0]"=w397:u16, "Registers[1]"=→"R101":u16, "Registers[2]"=→"R102":u16, "Registers[3]"=→"R103":u16, "Registers[4]"=→"R104":u16, "Registers[5]"=→"R105":u16, "Registers[6]"=→"R106":u16, "Registers[7]"=→"R107":u16, "Registers[8]"=→"R108":u16, "Registers[9]"=→"R109":u16, "Registers[10]"=→"R110":u16, "Registers[11]"=w394:u16, "Registers[12]"=→"R112":u16, "Registers[13]"=w392:u16, "Registers[16]"=→"R116":u16, "Registers[17]"=→"R117":u16, "Registers[18]"=w390:u16, "Registers[20]"=→"R120":u16, "Registers[21]"=→"R121":u16, "Registers[22]"=→"R122":u16, "Registers[23]"=→"R123":u16)  [unwired: 3 out]
            n223 = local write "R100"(w397) -> ()
            n224 = local write "R111"(w394) -> ()
            n225 = local write "R113"(w392) -> ()
            n226 = local write "R118"(w390) -> ()
          }
          frame "多个写入" {
            n227 = Unbundle By Name(w420) -> ("数据"=w419:variant)
            n228 = Variant To Data(type=T13 {"starting address"=0, "holding register values"=[]}, Variant=w419) -> (data=w417:T13)  [unwired: 1 in, 1 out]
            n229 = Unbundle By Name(w417) -> ("starting address"=w416:u16, "holding register values"=w415:u16[])
            n230 = call <vilib>:"Write Multiple Registers.vi"("error in (no error)"=w423, "values"=w415, "starting address"=w416, "MB session in"=w424) -> ("error out"=w422:errorcluster, "MB session out"=w421:refnum<class "MB_Master.lvclass">)  [unwired: 6 in]
          }
          frame "单个写入" {
            n231 = Unbundle By Name(w430) -> ("数据"=w429:variant)
            n232 = Variant To Data(type=T14 {"starting address"=0, "holding register value"=0}, Variant=w429) -> (data=w427:T14)  [unwired: 1 in, 1 out]
            n233 = Unbundle By Name(w427) -> ("starting address"=w426:u16, "holding register value"=w425:u16)
            n234 = call <vilib>:"Write Single Register.vi"("error in (no error)"=w433, "value"=w425, "address"=w426, "MB session in"=w434) -> ("error out"=w432:errorcluster, "MB session out"=w431:refnum<class "MB_Master.lvclass">)  [unwired: 6 in]
          }
          frame "线圈写入" {
            n235 = Unbundle By Name(w440) -> ("数据"=w439:variant)
            n236 = Variant To Data(type=T15 {"starting address"=0, "coil values"=[]}, Variant=w439) -> (data=w437:T15)  [unwired: 1 in, 1 out]
            n237 = Unbundle By Name(w437) -> ("starting address"=w436:u16, "coil values"=w435:bool[])
            n238 = call <vilib>:"Write Multiple Coils.vi"("error in (no error)"=w443, "values"=w435, "starting address"=w436, "MB session in"=w444) -> ("error out"=w442:errorcluster, "MB session out"=w441:refnum<class "MB_Master.lvclass">)  [unwired: 6 in]
          }
          frame "shutdown" {
            n239 = call <vilib>:"Write Single Register.vi"("error in (no error)"=w450, "value"=u16 0, "address"=u16 4047, "MB session in"=w454) -> ("error out"=w449:errorcluster, "MB session out"=w453:refnum<class "MB_Master.lvclass">)  [unwired: 6 in]
            n240 = call-dynamic "Close Session.vi"("error in (no error)"=w449, "MB session in"=w453) -> ("error out"=w455:errorcluster)  [unwired: 9 in]
            n241 = call "文件对话框"("start path"=path "D:/SRC") -> ("selected path"=w448:path, "cancelled"=w446:bool)  [unwired: 11 in, 2 out]
            n242 = call <vilib>:"Clear Errors.vi"("error in (no error)"=w455) -> ("error out"=w445:errorcluster)  [unwired: 5 in, 1 out]
            n243 = case shown="假" w446 {
              tunnel: w448 -> [w461 _]
              tunnel: w445 -> [_ _]
              frame False {
                n244 = Path To String(path=w461) -> (string=w458:string)
                n245 = Format Into String(format string="  - \"%s\"" ("格式字符串"), initial string="\"C:\\Program Files\\Fatek\\WinProladder\\WProlad.exe\"" ("command line"), w458) -> (resulting string=w459:string)  [unwired: 1 in, 1 out]
                n246 = call <vilib>:"System Exec.vi"("command line"=w459) -> ("error out"=w462:errorcluster)  [unwired: 7 in, 3 out]
                n247 = case shown="错误" w462 {
                  tunnel: w458 -> [_ w465]
                  frame No Error {
                  }
                  frame Error {
                    n248 = Format Into String(format string="  - \"%s\"" ("格式字符串"), initial string="\"C:\\Program Files (x86)\\Fatek\\WinProladder\\WProlad.exe\"" ("command line"), w465) -> (resulting string=w463:string)  [unwired: 1 in, 1 out]
                    n249 = call <vilib>:"System Exec.vi"("command line"=w463) -> ()  [unwired: 7 in, 4 out]
                  }
                }
              }
              frame True {
              }
            }
          }
        }
      }
      frame Error {
        n250 = Unbundle By Name(w471) -> ("code"=w473:i32)
        n251 = case shown="-1073807343" w473 {
          tunnel: w472 -> [w475 w479]
          tunnel: w471 -> [w474 w481]
          tunnel: [w474 w480] -> w469
          tunnel: [w475 w479] -> w470
          tunnel: w467 -> [_ w478]
          frame Default {
          }
          frame -1073807343 {
            n252 = Flush Queue(queue=w478) -> (queue out=w477:refnum<queue>)  [unwired: 1 in, 2 out]
            n253 = call-dynamic "Close Session.vi"("error in (no error)"=w481, "MB session in"=w479) -> ("error out"=w480:errorcluster)  [unwired: 9 in]
            n254 = disable-structure shown="禁用" {
              disable-tunnel: w477 -> [w482 _]
              frame Disabled {
                n255 = Enqueue Element At Opposite End(queue=w482, element=cluster{"命令":string, "数据":variant} {"命令"="init", "数据"=variant} ("元素")) -> ()  [unwired: 2 in, 3 out]
              }
              frame Enabled {
              }
            }
            n256 = Wait (ms)(milliseconds to wait=u32 2000 ("等待时间（毫秒）")) -> ()  [unwired: 1 out]
          }
        }
        n257 = call <vilib>:"Clear Errors.vi"("error in (no error)"=w469) -> ("error out"=w468:errorcluster)  [unwired: 5 in, 1 out]
      }
    }
    n258 = Unbundle By Name(w251) -> ("status"=→"通讯故障":bool)
  }
  n259 = property on="多列列表框" class="MCListbox (严格)"("ItemNames"=string[][] [["待机"], ["初始化"], ["水样润洗"], ["一级水样池进样"], ["二级水样池进样"], ["一级补充水样"], ["沉淀配水"], ["反冲洗"], ["采样池储水"], ["结束"]] ("项名")) -> ()  [unwired: 2 in, 2 out]
  n260 = call-dynamic "Close Session.vi"("error in (no error)"=w5, "MB session in"=w4) -> ()  [unwired: 9 in, 1 out]
